vi "main 0.8.vi"() -> ()   [LabVIEW 2012]
uses:
  coherent/CH_LM/CH_LM Communication Mode.ctl
  ISEGNHQxxu/iseg NHQ VISA Control.ctl
  <vilib>/Utility/file.llb/Read From Spreadsheet File (DBL).vi
  <vilib>/Analysis/1siggen.llb/Ramp Pattern by Samples.vi
  <vilib>/Utility/file.llb/Write To Spreadsheet File (DBL).vi
  <vilib>/Utility/file.llb/Write To Spreadsheet File (string).vi
  <vilib>/Platform/browser.llb/Open URL in Default Browser (path).vi
  <vilib>/Analysis/NI_AALBase.lvlib
  coherent/CH_LM.lvlib
panel:
  out "x-y":u32
  in  "avg[t] acc[f]":bool=TRUE
  in  "frames":i32=1000
  in  "array size 2":i32
  in  "dark_load":bool
  in  "binning":dbl=4.0
  in  "exp time [s]":dbl=0.01
  in  "threshold":i32=110
  in  "dark?":bool=TRUE
  in  "count?":bool
  in  "array size":i32
  out "power noise-o-meter":dbl format="%.1g"
  out "signal noise-o-meter":dbl format="%.1g"
  in  "Nominal Voltage":sgl=50.0 max=4000 format="%.2f"
  in  "volt_set":bool
  in  "open base path":bool
  out "laser power":sgl[unit]=6.5658234e-09 format="%.3f"
  out "Actual Voltage":dbl[unit]=-50.050000000000004 format="%.2f"
  out "Waveform Chart":dbl(graph)
  in  "Path":path=path "Y:/Ediff/data/2016/10/161018"
  in  "stop":bool
  out "Slide":dbl(slide)=0.999 scale=0.0..1.0
  in  "Tab Control":T1(tab)
  in  "snap":bool
  in  "dark":bool
  in  "savebin":bool
  in  "savepng":bool
  out "meas_voltage":i32
  in  "header":string="PowerVoltScan1"
  in  "meas_start_power":bool
  out "meas_power":sgl[unit]=6.5658234e-09 format="%.3f"
  out "Slide 2":dbl(slide)=0.999 scale=0.0..1.0
  in  "meas_stop_volt":bool
  in  "meas_start_volt":bool
  in  "head":string="PowerVoltScan1"
  in  "volt_start":dbl format="%0.2f"
  in  "volt_end":dbl=1.0 format="%0.2f"
  in  "volt_samples":i32=128
  in  "move2com":bool
  in  "window2":dbl=10000.0 caption="+/- window" format="%#_6e"
  in  "steps2":u32=21 caption="steps"
  out "XY":dbl[][](graph)
  in  "meas_start_XY":bool
  in  "Axis2":string(combo)="4D Z"
  in  "Axis1":string(combo)="4D Z"
  in  "window1":dbl=10000.0 caption="+/- window" format="%#_6e"
  in  "steps1":u32=21 caption="steps"
  in  "meas_stop_XY":bool
  in  "showcom":bool
  in  "VISA ISEG":refnum<visa-resource-name>="COM6"
  in  "Channel (A)":enum16{"A", "B"}(ring)=enum."B"
  in  "IP address":string="172.24.192.135"
  out "error out":errorcluster
  out "coherent":errorcluster
  in  "volt_timeout":u32=6000
  in  "volt_threshold":sgl=2.0 max=4000 format="%.2f"
  out "captured":dbl[][](graph)
  out "live":dbl[][](graph)
  in  "close":bool
  # "%"
  # "Axis2"
  # "Axis1"
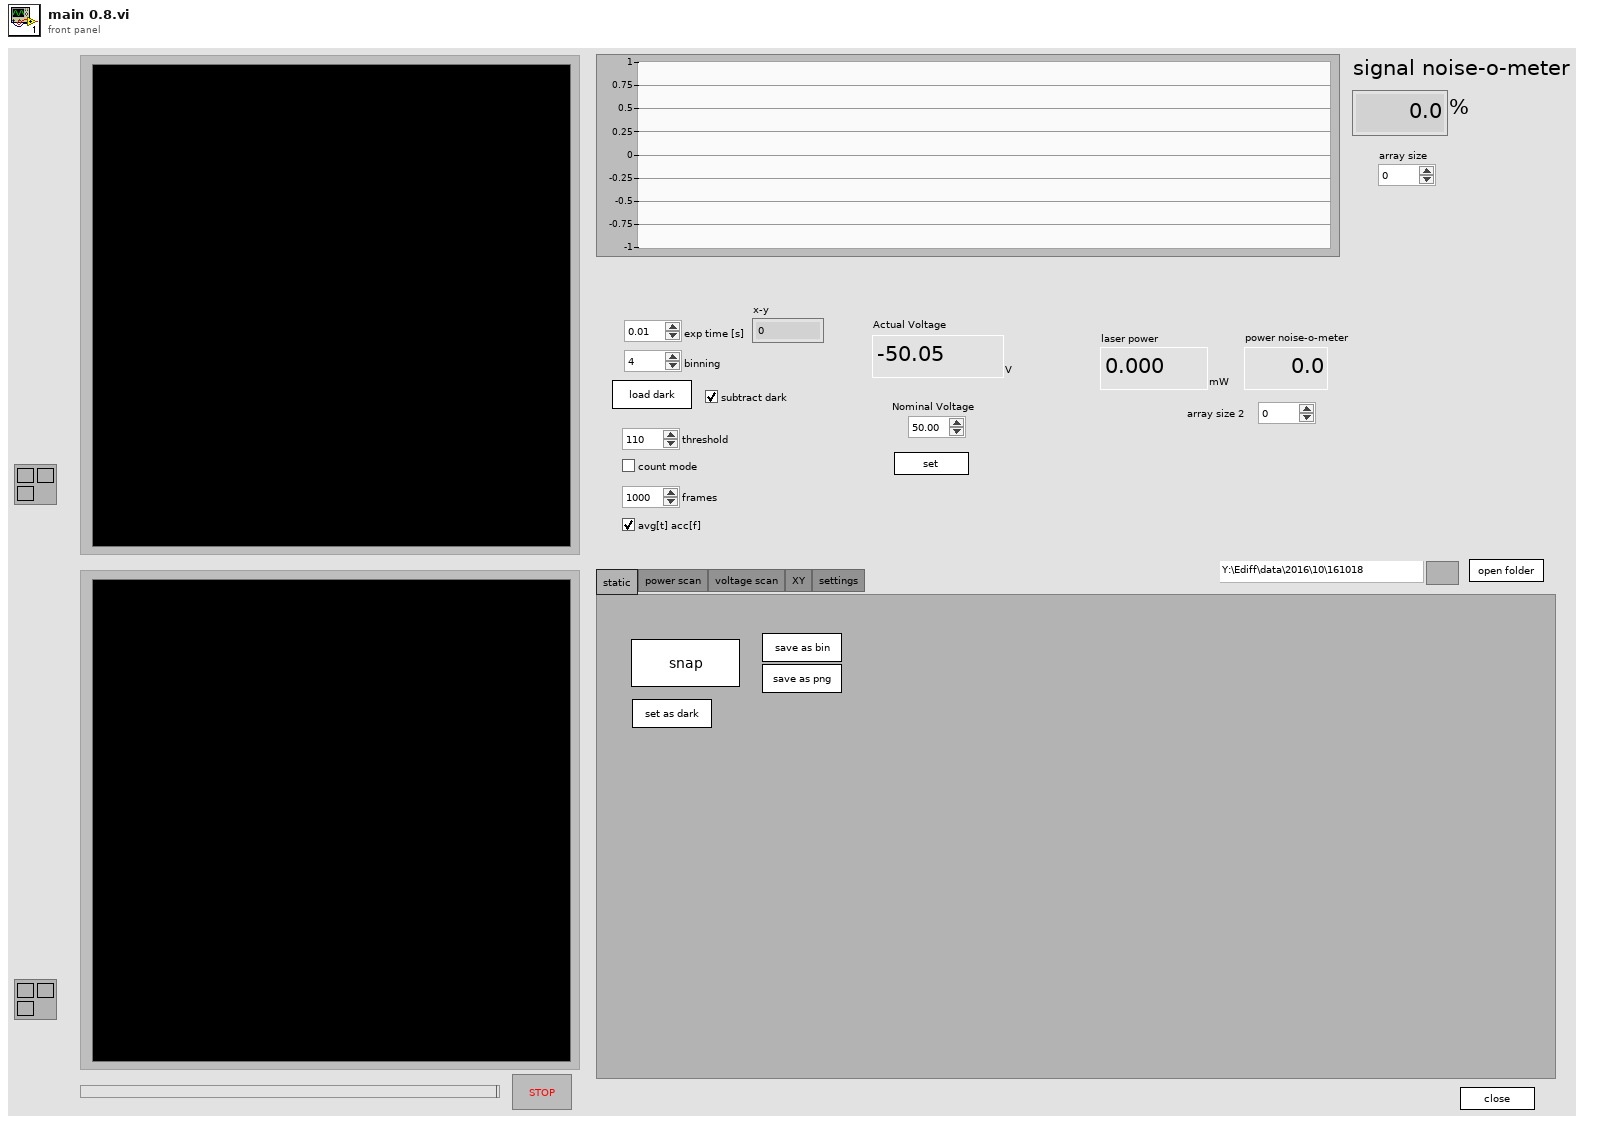
[diagram p1: front panel]
types:
  T1 = enum32{"static", "power scan", "voltage scan", "XY", "settings"}
  T2 = typedef "CH_LM.lvlib/CH_LM Communication Mode.ctl" = enum16{"None", "USB", "GPIB", "RS232"}
  T3 = typedef "Image Type" = u32
  T4 = typedef "IMAQ Image.ctl" = refnum<image>
  T5 = cluster{"height":u32, "width":u32, "datatype":u32}
  T6 = typedef "iseg NHQ VISA Control.ctl" = cluster{"VISA Resource Name":refnum<visa-resource-name>, "FP Notation":bool, "Maximum Voltage":u32, "Maximum Current":u32}
  T7 = typedef "CH_LM.lvlib/CH_LM Streaming Data.ctl" = cluster{"Value":sgl, "Quad Distance":cluster{"X":sgl, "Y":sgl}, "Display Data":cluster{"Format ID":u8, "Scale ID":u8}, "Unit ID":u8, "Flags":u32, "Pulse Period":u32, "Sequence ID":u32, "Unit String":string}
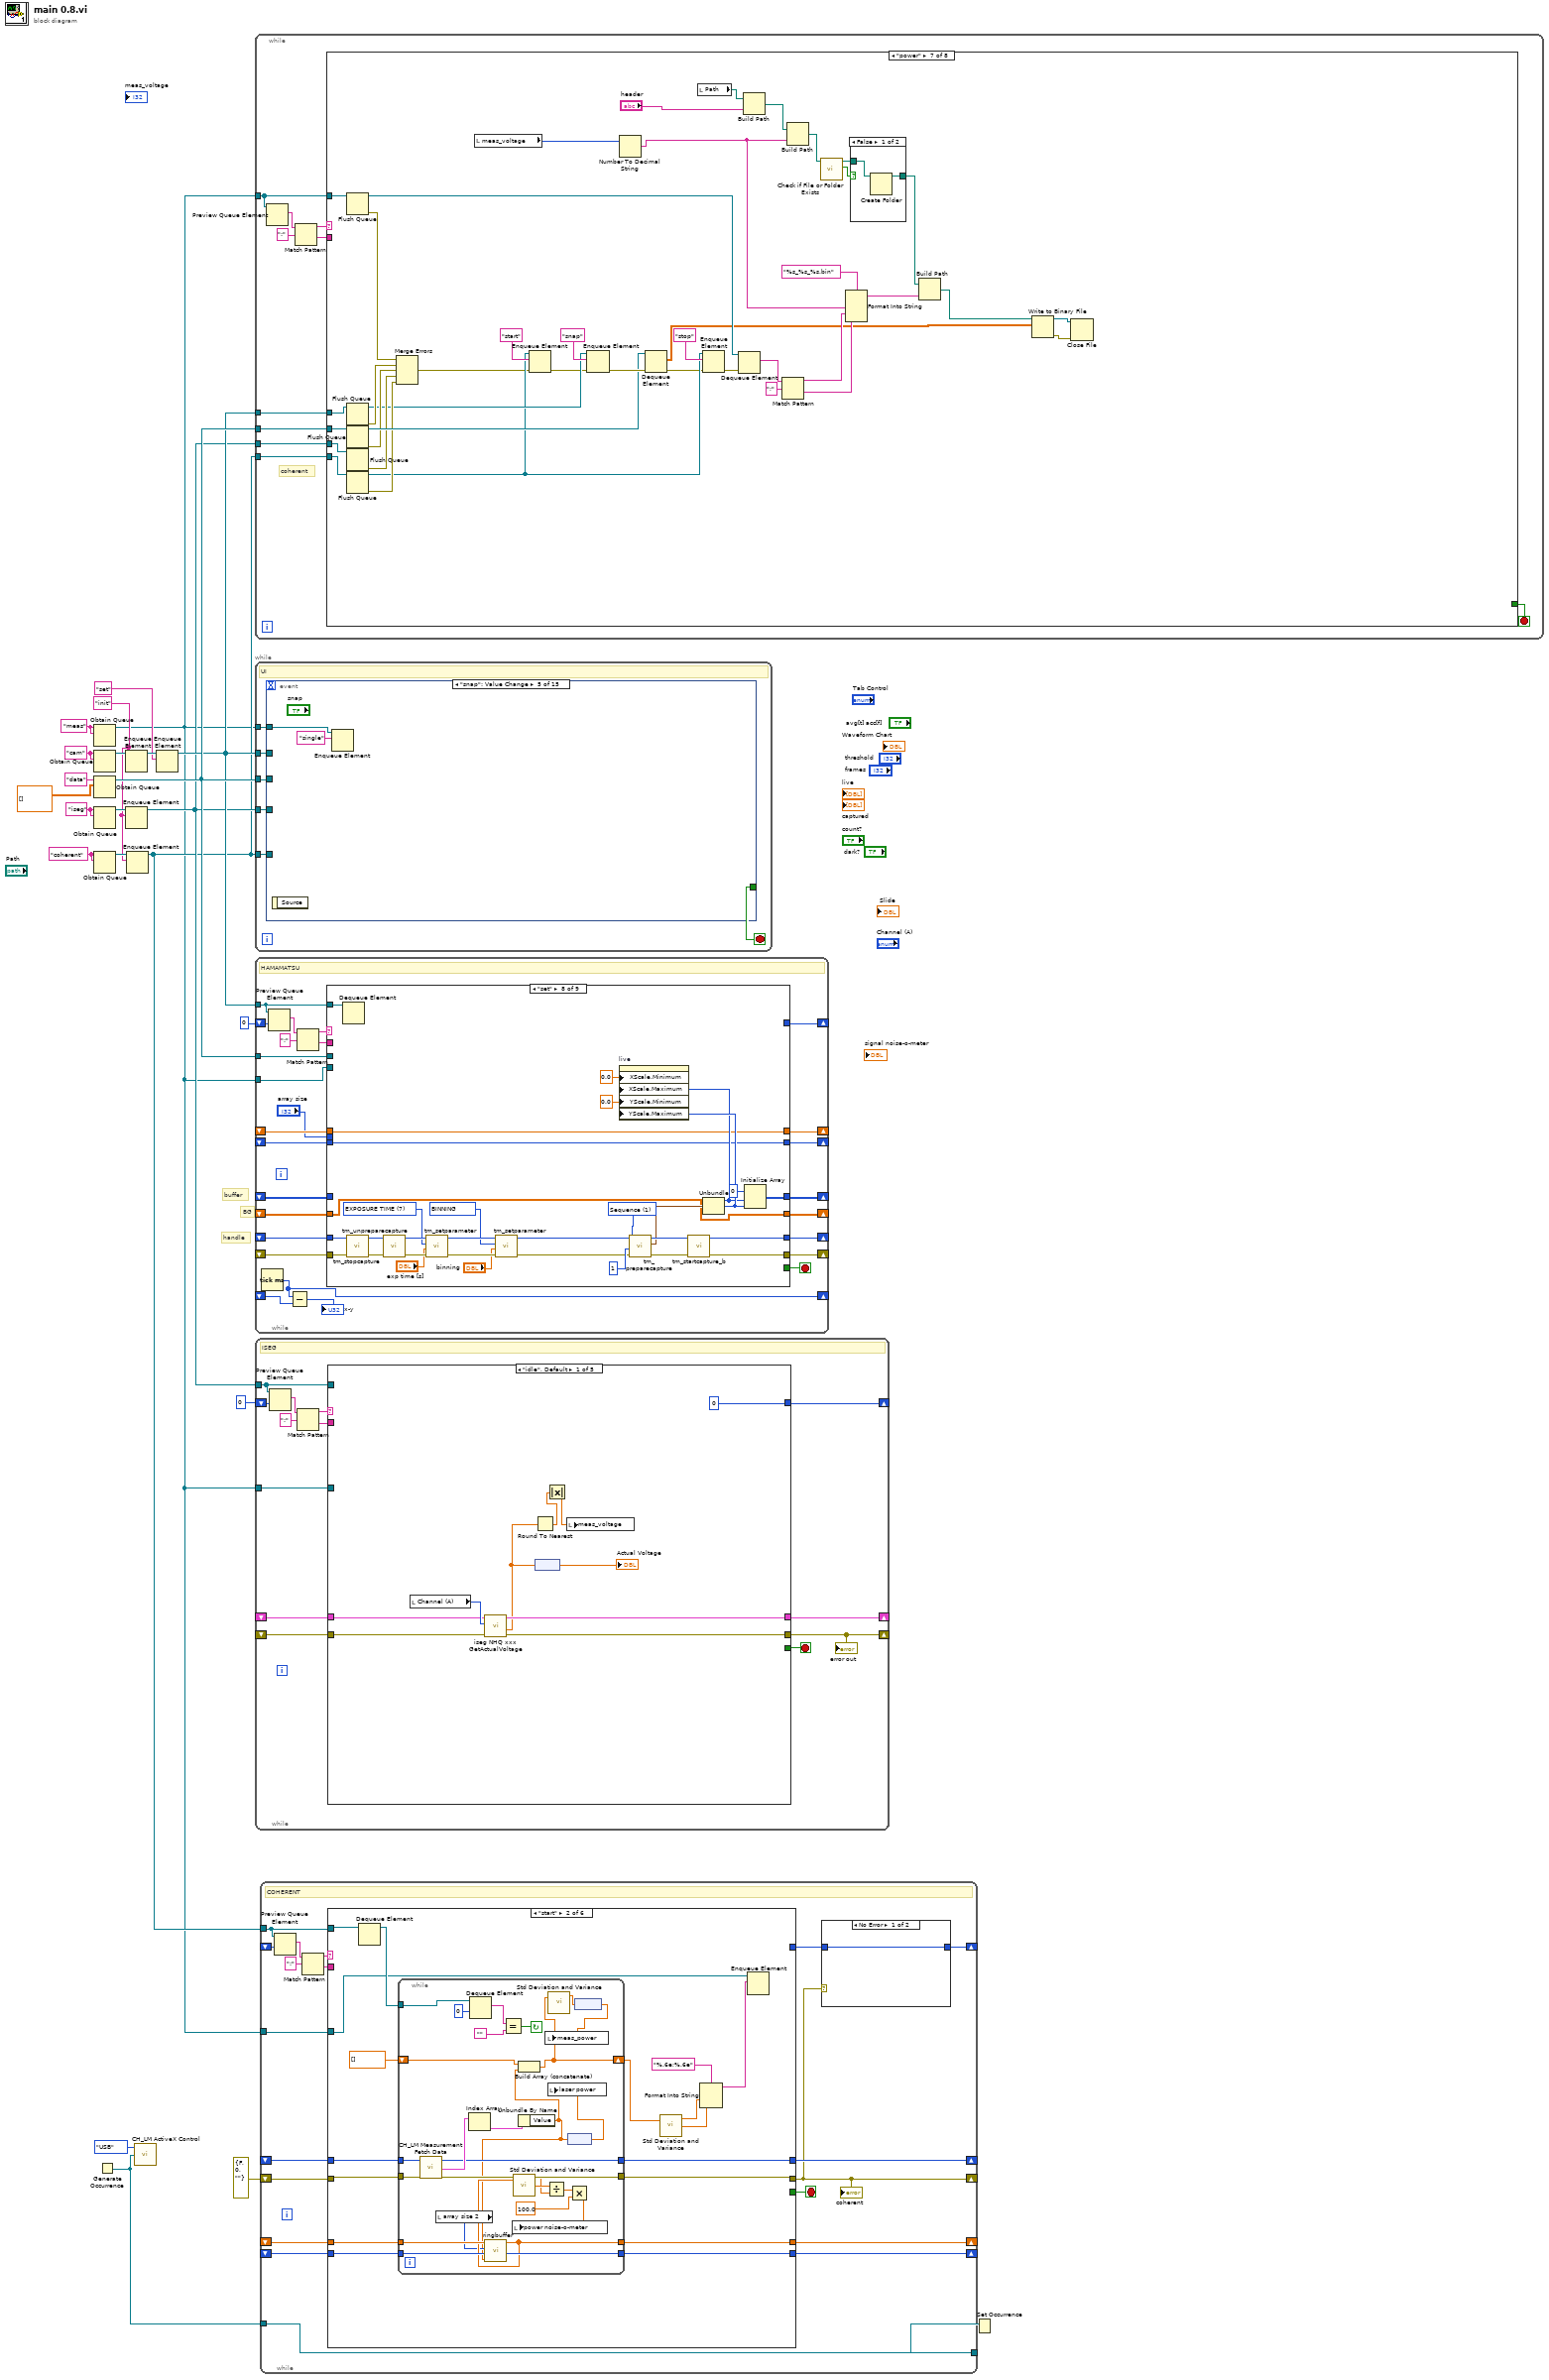
[diagram p0: block diagram]
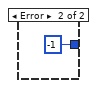
[diagram p2: hidden frame]
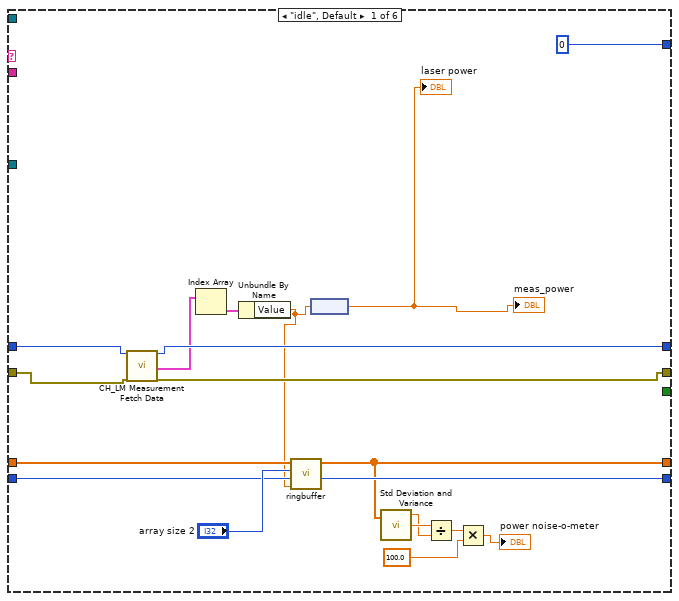
[diagram p3: hidden frame]
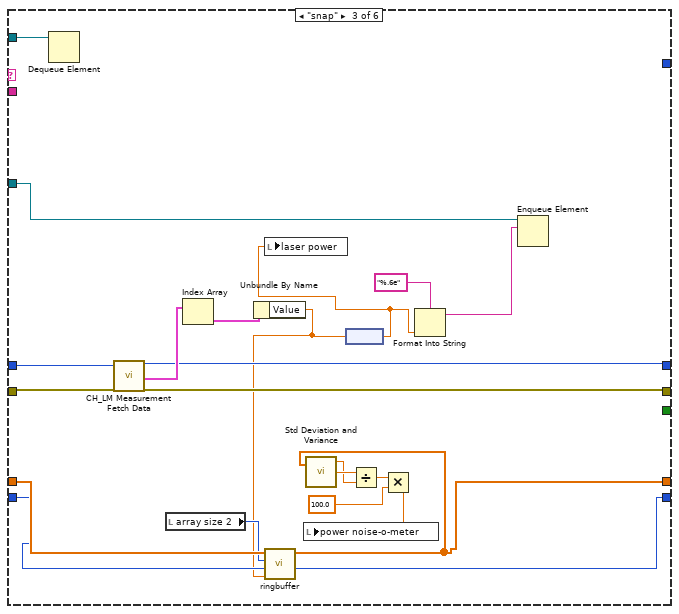
[diagram p4: hidden frame]
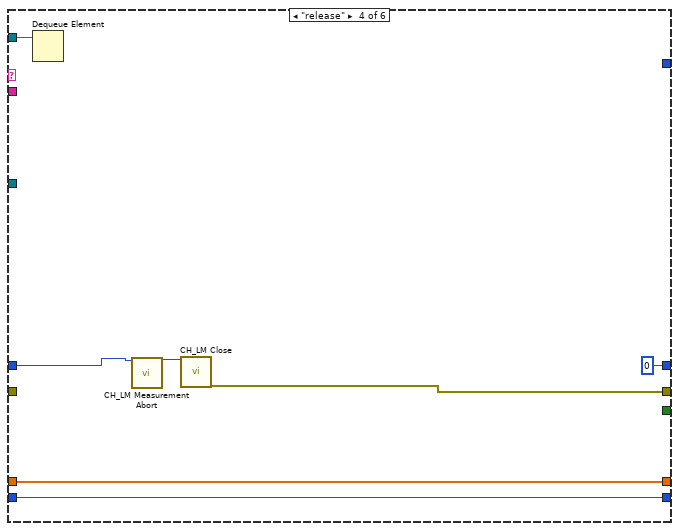
[diagram p5: hidden frame]
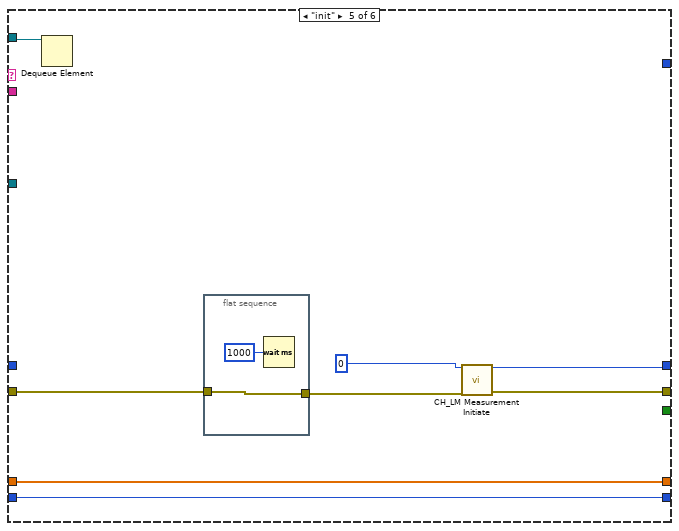
[diagram p6: hidden frame]
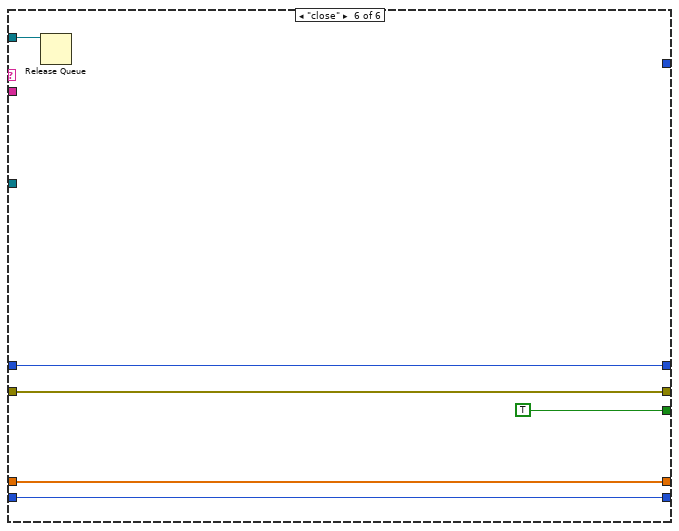
[diagram p7: hidden frame]
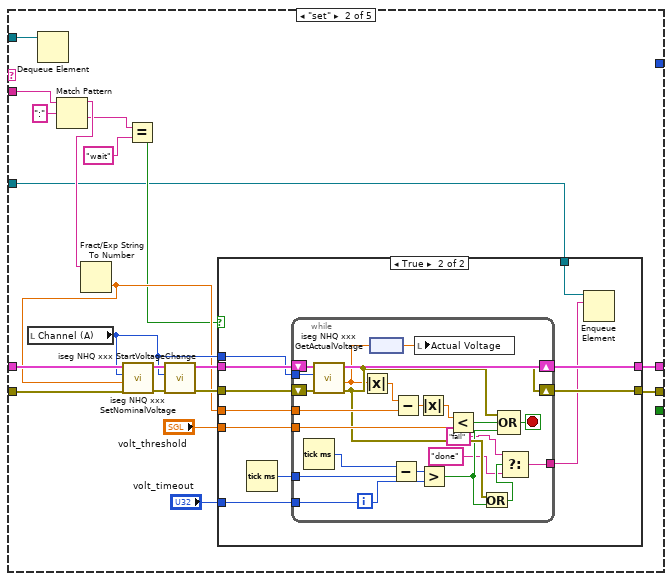
[diagram p8: hidden frame]
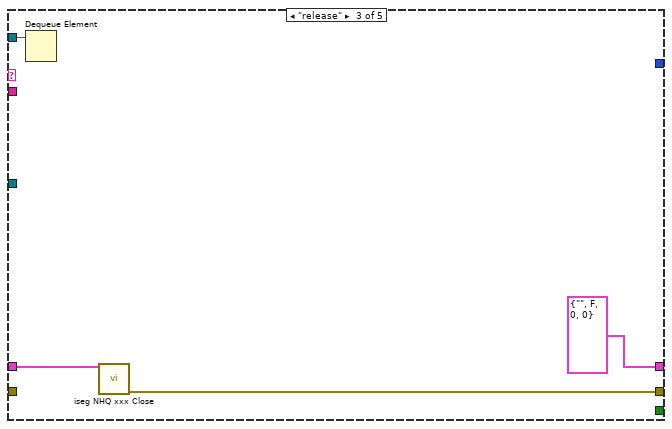
[diagram p10: hidden frame]
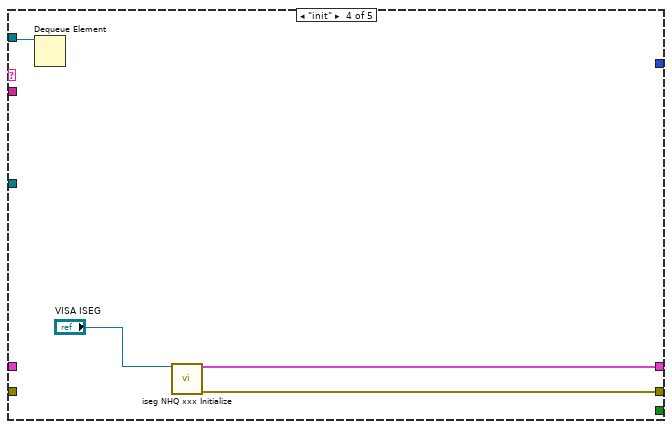
[diagram p11: hidden frame]
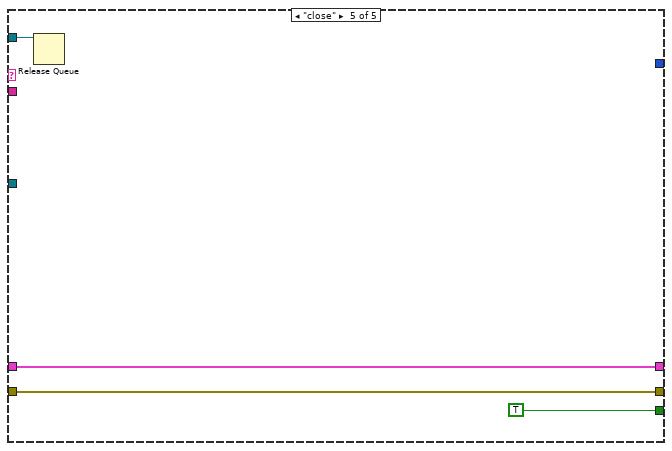
[diagram p12: hidden frame]
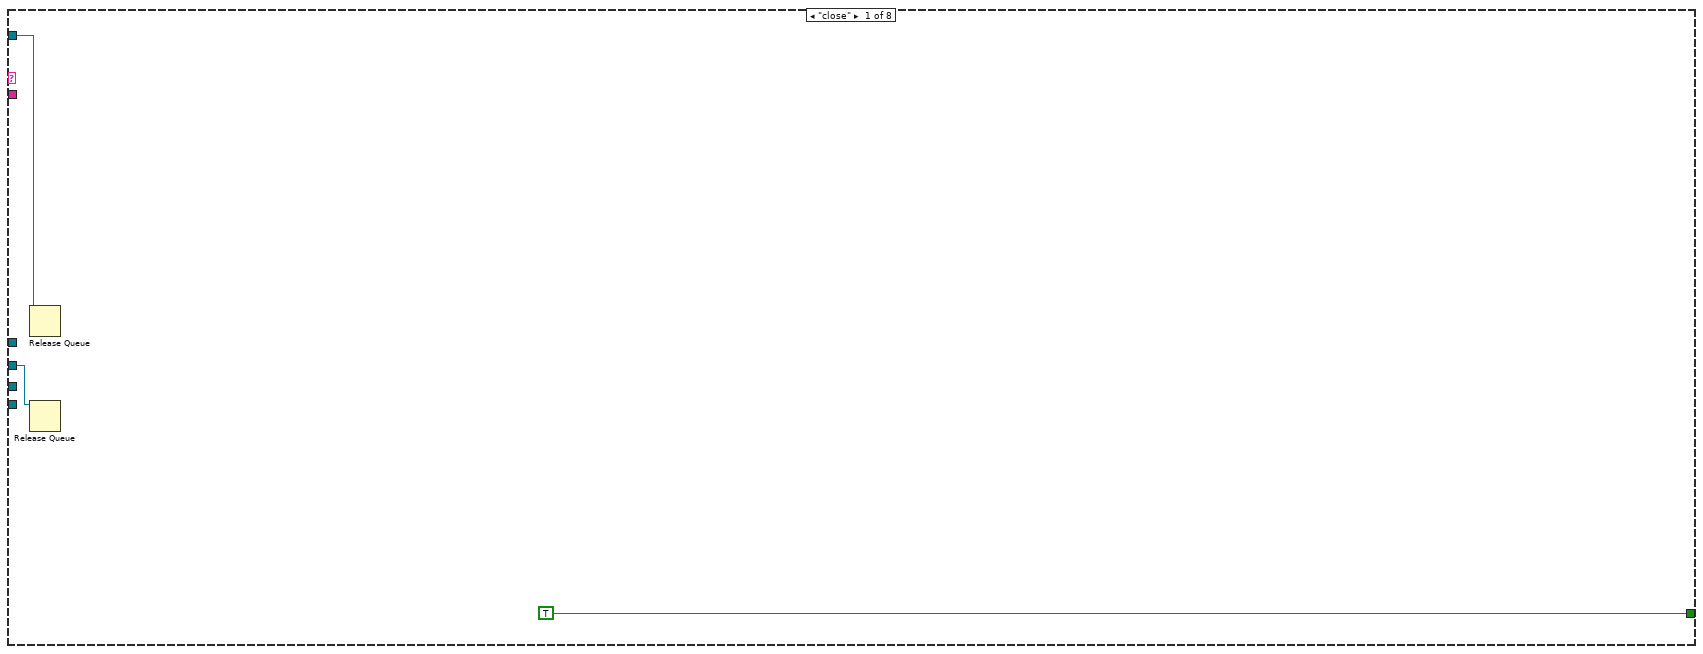
[diagram p13: hidden frame]
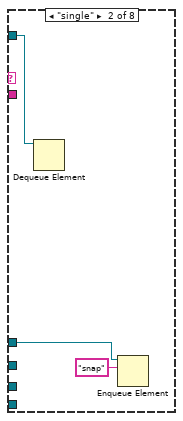
[diagram p14: hidden frame]
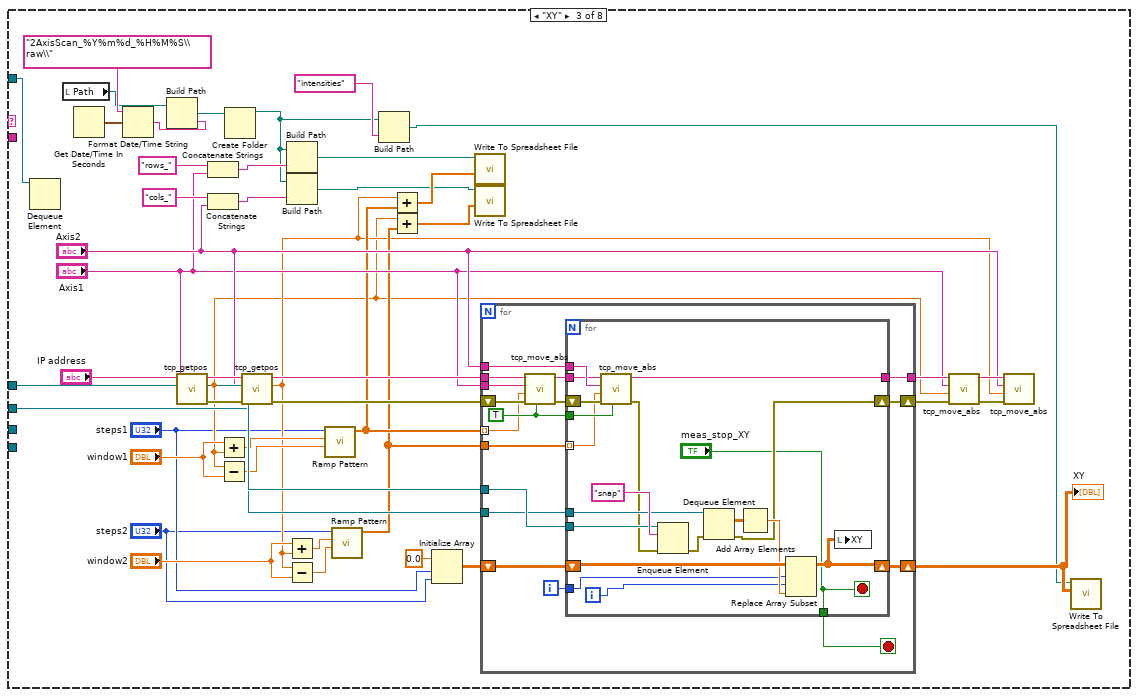
[diagram p15: hidden frame]
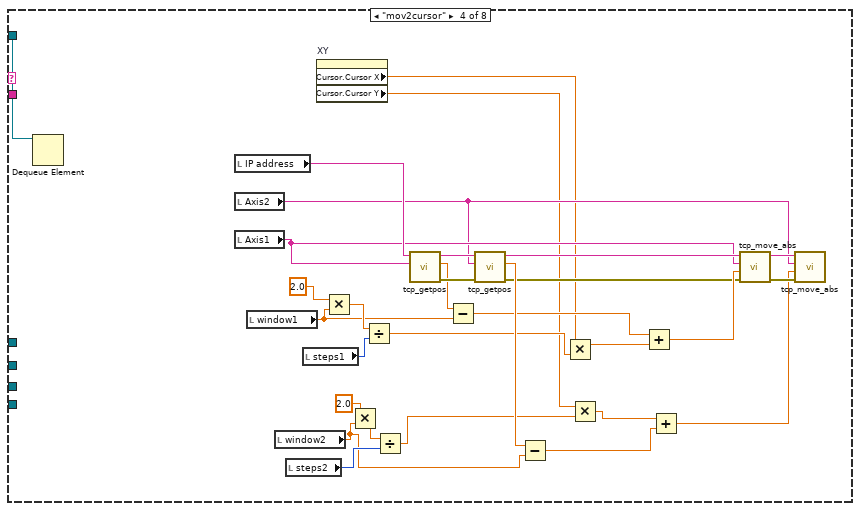
[diagram p16: hidden frame]
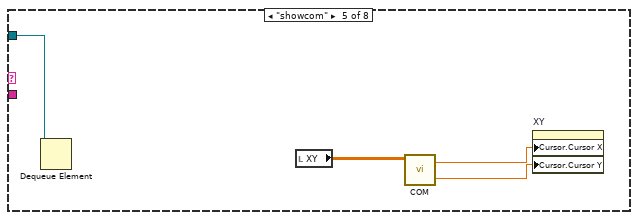
[diagram p17: hidden frame]
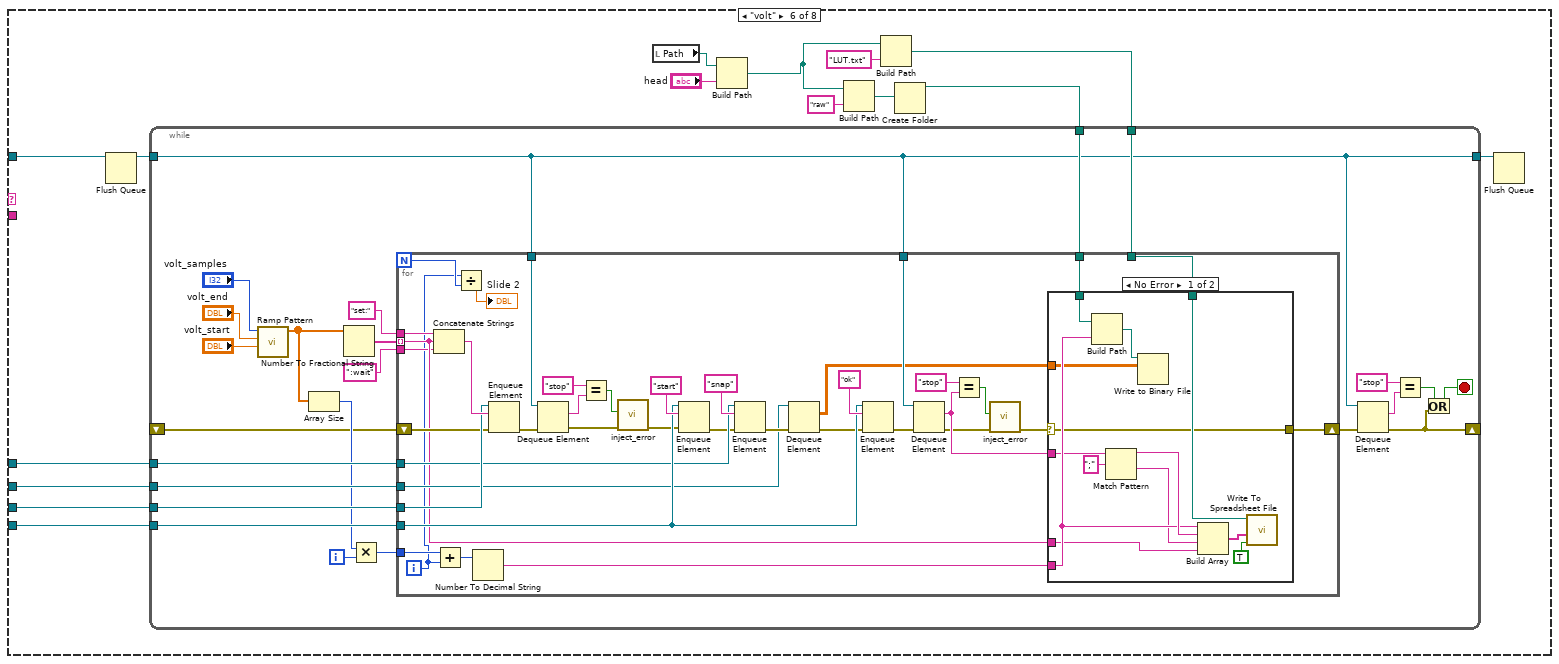
[diagram p18: hidden frame]
diagram:
  w8 = "coherent" ("name (unnamed)")
  w13 = "iseg" ("name (unnamed)")
  w7 = "init" ("element")
  w20 = "meas" ("name (unnamed)")
  w21 = "cam" ("name (unnamed)")
  # "BG"
  # "handle"
  # "buffer"
  n1 = Obtain Queue(name (unnamed)=w20, element data type=w20) -> (queue out=w1:refnum<queue>)  [unwired: 3 in, 2 out]
  n2 = Obtain Queue(name (unnamed)=w21, element data type=w21) -> (queue out=w23:refnum<queue>)  [unwired: 3 in, 2 out]
  n3 = Obtain Queue(name (unnamed)=w13, element data type=w13) -> (queue out=w12:refnum<queue>)  [unwired: 3 in, 2 out]
  n4 = Obtain Queue(name (unnamed)="data", element data type=dbl[][] []) -> (queue out=w16:refnum<queue>)  [unwired: 3 in, 2 out]
  n5 = Obtain Queue(name (unnamed)=w8, element data type=w8) -> (queue out=w9:refnum<queue>)  [unwired: 3 in, 2 out]
  n6 = Generate Occurrence() -> (w5:refnum<k4>)
  n7 = Enqueue Element(queue=w23, element=w7) -> (queue out=w19:refnum<queue>)  [unwired: 2 in, 2 out]
  n8 = Enqueue Element(queue=w12, element=w7) -> (queue out=w10:refnum<queue>)  [unwired: 2 in, 2 out]
  n9 = Enqueue Element(queue=w9, element=w7) -> (queue out=w3:refnum<queue>)  [unwired: 2 in, 2 out]
  n10 = call "CH_LM ActiveX Control.vi"("Communication Mode"=CH_LM_Communication_Mode."USB", "MonitorStop Occurrence"=w5) -> ()  [unwired: 3 in, 1 out]
  n11 = Enqueue Element(queue=w19, element="set") -> (queue out=w15:refnum<queue>)  [unwired: 2 in, 2 out]
  n12 = while {
    tunnel: w1 -> [w29]
    tunnel: w16 -> [w28]
    tunnel: w15 -> [w26]
    tunnel: w10 -> [w25]
    tunnel: w3 -> [w24]
    stop <- w27 stop-if-true
    # "coherent"
    n13 = Preview Queue Element(queue=w29) -> (element=w33:string)  [unwired: 2 in, 3 out]
    n14 = Match Pattern(string=w33, regular expression=":") -> (before substring=w31:string, after substring=w30:string)  [unwired: 1 in, 2 out]
    n15 = case shown="\"power\"" w31 {
      tunnel: w30 -> [_ _ _ _ _ _ _ _]
      tunnel: w29 -> [w35 w39 w84 w150 w151 w169 w285 _]
      tunnel: w28 -> [w36 _ w80 _ _ w161 w281 _]
      tunnel: [TRUE _ _ _ _ _ _ _] -> w27
      tunnel: w26 -> [_ w38 w81 _ _ w162 w279 _]
      tunnel: w25 -> [_ _ _ _ _ w163 w278 _]
      tunnel: w24 -> [_ _ _ _ _ w164 w277 _]
      frame "close" {
        n16 = Release Queue(queue=w35) -> ()  [unwired: 2 in, 3 out]
        n17 = Release Queue(queue=w36) -> ()  [unwired: 2 in, 3 out]
      }
      frame "single" {
        n18 = Dequeue Element(queue=w39) -> ()  [unwired: 2 in, 4 out]
        n19 = Enqueue Element(queue=w38, element="snap") -> ()  [unwired: 2 in, 3 out]
      }
      frame "XY" {
        n20 = Dequeue Element(queue=w84) -> ()  [unwired: 2 in, 4 out]
        n21 = local read "Path"() -> (w75:path)
        n22 = Get Date/Time In Seconds() -> (seconds since 1Jan1904=w79:timestamp)
        n23 = Format Date/Time String(time format string (%c)="2AxisScan_%Y%m%d_%H%M%S\\raw\\", seconds (now)=w79) -> (date/time string=w43:string)  [unwired: 1 in]
        n24 = Build Path(base path=w75, name or relative path=w43) -> (appended path=w47:path)
        n25 = call "tcp_getpos.vi"("Axis"="Axis1", "IP address"="IP address") -> ("error out"=w76:errorcluster, "position"=w52:dbl, "IP address out"=w77:string)  [unwired: 7 in]
        n26 = Concatenate Strings("rows_" ("string"), "Axis1") -> (w44:string)
        n27 = Concatenate Strings("cols_" ("string"), "Axis2") -> (w74:string)
        n28 = Add(x="window1", y=w52) -> (x+y=w59:dbl)
        n29 = Subtract(x=w52, y="window1") -> (x-y=w58:dbl)
        n30 = Create Folder(path (use dialog)=w47) -> (created path=w42:path)  [unwired: 2 in, 2 out]
        n31 = call "tcp_getpos.vi"("error in (no error)"=w76, "Axis"="Axis2", "IP address"=w77) -> ("error out"=w69:errorcluster, "position"=w53:dbl, "IP address out"=w64:string)  [unwired: 6 in]
        n32 = Build Path(base path=w42, name or relative path=w44) -> (appended path=w41:path)
        n33 = Build Path(base path=w42, name or relative path=w74) -> (appended path=w40:path)
        n34 = Add(x="window2", y=w53) -> (x+y=w56:dbl)
        n35 = Subtract(x=w53, y="window2") -> (x-y=w57:dbl)
        n36 = call-poly <vilib>:"Ramp Pattern.vi"("start"=w58, "end"=w59, "samples"="steps1") -> ("Ramp Pattern"=w55:dbl[])  [unwired: 7 in, 1 out]
        n37 = call-poly <vilib>:"Ramp Pattern.vi"("start"=w57, "end"=w56, "samples"="steps2") -> ("Ramp Pattern"=w54:dbl[])  [unwired: 7 in, 1 out]
        n38 = Build Path(base path=w42, name or relative path="intensities") -> (appended path=w45:path)
        n39 = Add(x=w53, y=w55) -> (x+y=w51:dbl[])
        n40 = Add(x=w52, y=w54) -> (x+y=w50:dbl[])
        n41 = Initialize Array(0.0 ("element"), "steps1", "steps2") -> (w82:dbl[][])
        n42 = call-poly <vilib>:"Write To Spreadsheet File.vi"("1D data"=w51, "file path (dialog if empty)"=w41) -> ()  [unwired: 6 in, 1 out]
        n43 = call-poly <vilib>:"Write To Spreadsheet File.vi"("1D data"=w50, "file path (dialog if empty)"=w40) -> ()  [unwired: 6 in, 1 out]
        n44 = for {
          tunnel: "Axis1" -> [w101]
          tunnel: w81 -> [w100]
          tunnel: w80 -> [w99]
          tunnel: "Axis2" -> [w95]
          shift-right: [w94] -> w73
          shift-left: w82 -> [w98]
          shift-right: [w91] -> w70
          shift-left: w69 -> [w90]
          tunnel: [w88] -> w65
          tunnel: w64 -> [w87]
          tunnel: w55 -> [w85] mode=indexing
          tunnel: w54 -> [w86]
          i -> [w97]
          stop <- w89 stop-if-true
          w96 = TRUE ("wait4motiondone")
          n45 = call "tcp_move_abs.vi"("wait4motiondone"=w96, "error in (no error)"=w90, "destination nm/u°"=w85, "Axis"=w101, "IP address"=w87) -> ("error out"=w93:errorcluster, "IP address out"=w92:string)  [unwired: 4 in, 1 out]
          n46 = for {
            tunnel: w100 -> [w118]
            tunnel: w99 -> [w117]
            tunnel: w97 -> [w103]
            shift-right: [w108] -> w94
            shift-left: w98 -> [w116]
            tunnel: w96 -> [w112]
            tunnel: w95 -> [w111]
            tunnel: w92 -> [w109]
            shift-right: [w107] -> w91
            shift-left: w93 -> [w110]
            tunnel: ["meas_stop_XY"] -> w89
            tunnel: [w105] -> w88
            tunnel: w86 -> [w104] mode=indexing
            i -> [w102]
            stop <- "meas_stop_XY" stop-if-true
            n47 = call "tcp_move_abs.vi"("wait4motiondone"=w112, "error in (no error)"=w110, "destination nm/u°"=w104, "Axis"=w111, "IP address"=w109) -> ("error out"=w113:errorcluster, "IP address out"=w105:string)  [unwired: 4 in, 1 out]
            n48 = Enqueue Element(queue=w118, element="snap", error in (no error)=w113) -> (error out=w119:errorcluster)  [unwired: 1 in, 2 out]
            n49 = Dequeue Element(queue=w117, error in (no error)=w119) -> (element=w115:dbl[][], error out=w107:errorcluster)  [unwired: 1 in, 2 out]
            n50 = Add Array Elements(numeric array=w115) -> (sum=w114:dbl)
            n51 = Replace Array Subset(array=w116, new element=w114, index (row)=w103, index (col)=w102) -> (w108:dbl[][])
            n52 = local write "XY"(w108) -> ()
          }
        }
        "XY" <- w73
        n53 = call "tcp_move_abs.vi"("error in (no error)"=w70, "destination nm/u°"=w52, "Axis"="Axis1", "IP address"=w65) -> ("error out"=w72:errorcluster, "IP address out"=w71:string)  [unwired: 5 in, 1 out]
        n54 = call "tcp_move_abs.vi"("error in (no error)"=w72, "destination nm/u°"=w53, "Axis"="Axis2", "IP address"=w71) -> ()  [unwired: 5 in, 3 out]
        n55 = call-poly <vilib>:"Write To Spreadsheet File.vi"("2D data"=w73, "file path (dialog if empty)"=w45) -> ()  [unwired: 6 in, 1 out]
      }
      frame "mov2cursor" {
        n56 = Dequeue Element(queue=w150) -> ()  [unwired: 2 in, 4 out]
        n57 = local read "IP address"() -> (w145:string)
        n58 = local read "Axis2"() -> (w123:string)
        n59 = local read "Axis1"() -> (w124:string)
        n60 = local read "window1"() -> (w138:dbl)
        n61 = local read "window2"() -> (w137:dbl)
        n62 = local read "steps2"() -> (w143:u32)
        n63 = local read "steps1"() -> (w144:u32)
        n64 = property on="XY" class="IntGraph (strict)"() -> ("Cursor.Cursor X"=w122:dbl, "Cursor.Cursor Y"=w121:dbl)  [unwired: 2 in, 2 out]
        n65 = Multiply(x=2.0, y=w138) -> (x*y=w142:dbl)
        n66 = Multiply(x=2.0, y=w137) -> (x*y=w139:dbl)
        n67 = Divide(x=w142, y=w144) -> (x/y=w136:dbl)
        n68 = Divide(x=w139, y=w143) -> (x/y=w133:dbl)
        n69 = call "tcp_getpos.vi"("Axis"=w124, "IP address"=w145) -> ("error out"=w148:errorcluster, "position"=w146:dbl, "IP address out"=w149:string)  [unwired: 7 in]
        n70 = Subtract(x=w146, y=w138) -> (x-y=w134:dbl)
        n71 = call "tcp_getpos.vi"("error in (no error)"=w148, "Axis"=w123, "IP address"=w149) -> ("error out"=w126:errorcluster, "position"=w147:dbl, "IP address out"=w125:string)  [unwired: 6 in]
        n72 = Subtract(x=w147, y=w137) -> (x-y=w131:dbl)
        n73 = Multiply(x=w122, y=w136) -> (x*y=w135:dbl)
        n74 = Multiply(x=w121, y=w133) -> (x*y=w132:dbl)
        n75 = Add(x=w134, y=w135) -> (x+y=w128:dbl)
        n76 = Add(x=w132, y=w131) -> (x+y=w127:dbl)
        n77 = call "tcp_move_abs.vi"("error in (no error)"=w126, "destination nm/u°"=w128, "Axis"=w124, "IP address"=w125) -> ("error out"=w130:errorcluster, "IP address out"=w129:string)  [unwired: 5 in, 1 out]
        n78 = call "tcp_move_abs.vi"("error in (no error)"=w130, "destination nm/u°"=w127, "Axis"=w123, "IP address"=w129) -> ()  [unwired: 5 in, 3 out]
      }
      frame "showcom" {
        n79 = Dequeue Element(queue=w151) -> ()  [unwired: 2 in, 4 out]
        n80 = local read "XY"() -> (w154:dbl[][])
        n81 = call "COM.vi"("Array"=w154) -> ("Y out"=w152:dbl, "X out"=w153:dbl)  [unwired: 3 in]
        n82 = property on="XY" class="IntGraph (strict)"("Cursor.Cursor X"=w153, "Cursor.Cursor Y"=w152) -> ()  [unwired: 2 in, 2 out]
      }
      frame "volt" {
        n83 = Flush Queue(queue=w169) -> (queue out=w165:refnum<queue>)  [unwired: 1 in, 2 out]
        n84 = local read "Path"() -> (w168:path)
        n85 = Build Path(base path=w168, name or relative path="head") -> (appended path=w156:path)
        n86 = Build Path(base path=w156, name or relative path="raw") -> (appended path=w158:path)
        n87 = Build Path(base path=w156, name or relative path="LUT.txt") -> (appended path=w159:path)
        n88 = Create Folder(path (use dialog)=w158) -> (created path=w157:path)  [unwired: 2 in, 2 out]
        n89 = while {
          tunnel: w165 -> [w170]
          tunnel: w164 -> [w193]
          tunnel: w163 -> [w187]
          tunnel: w162 -> [w186]
          tunnel: w161 -> [w185]
          tunnel: w159 -> [w180]
          tunnel: w157 -> [w179]
          shift-right: [w172] -> _
          shift-left: _ -> [w177]
          tunnel: [w170] -> w155
          i -> [w184]
          stop <- w171 stop-if-true
          n90 = call-poly <vilib>:"Ramp Pattern.vi"("start"="volt_start", "end"="volt_end", "samples"="volt_samples") -> ("Ramp Pattern"=w183:dbl[])  [unwired: 7 in, 1 out]
          n91 = Array Size(array=w183) -> (size(s)=w182:i32)
          n92 = Number To Fractional String(number=w183) -> (F-format string=w189:string[])  [unwired: 3 in]
          n93 = Multiply(x=w182, y=w184) -> (x*y=w181:i32)
          n94 = for {
            N -> [w196]
            tunnel: w193 -> [w223]
            tunnel: w170 -> [w230]
            tunnel: w189 -> [w213] mode=indexing
            tunnel: "set:" ("element") -> [w227]
            tunnel: w187 -> [w226]
            tunnel: w170 -> [w224]
            tunnel: w186 -> [w221]
            tunnel: w185 -> [w218]
            shift-right: [w198] -> w178
            shift-left: w177 -> [w216]
            tunnel: w181 -> [w215]
            tunnel: w180 -> [w212]
            tunnel: w179 -> [w211]
            tunnel: ":wait" ("element") -> [w197]
            i -> [w195]
            n95 = Concatenate Strings(w227, w213, w197) -> (w228:string)
            n96 = Add(x=w215, y=w195) -> (x+y=w214:i32)
            n97 = Divide(x=w195, y=w196) -> (x/y=→"Slide 2":dbl)
            n98 = Number To Decimal String(number=w214) -> (decimal integer string=w210:string)  [unwired: 1 in]
            n99 = Enqueue Element(queue=w226, element=w228, error in (no error)=w216) -> (error out=w225:errorcluster)  [unwired: 1 in, 2 out]
            n100 = Dequeue Element(queue=w224, error in (no error)=w225) -> (element=w207:string, error out=w205:errorcluster)  [unwired: 1 in, 2 out]
            n101 = Equal?(x="stop" ("y"), y=w207) -> (x = y?=w204:bool)
            n102 = call "inject_error.vi"("error in"=w205, "s"=w204) -> ("error out"=w206:errorcluster)  [unwired: 9 in]
            n103 = Enqueue Element(queue=w223, element="start", error in (no error)=w206) -> (error out=w220:errorcluster)  [unwired: 1 in, 2 out]
            n104 = Enqueue Element(queue=w221, element="snap", error in (no error)=w220) -> (error out=w219:errorcluster)  [unwired: 1 in, 2 out]
            n105 = Dequeue Element(queue=w218, error in (no error)=w219) -> (element=w209:dbl[][], error out=w217:errorcluster)  [unwired: 1 in, 2 out]
            n106 = Enqueue Element(queue=w223, element="ok", error in (no error)=w217) -> (error out=w229:errorcluster)  [unwired: 1 in, 2 out]
            n107 = Dequeue Element(queue=w230, error in (no error)=w229) -> (element=w201:string, error out=w200:errorcluster)  [unwired: 1 in, 2 out]
            n108 = Equal?(x="stop" ("y"), y=w201) -> (x = y?=w203:bool)
            n109 = call "inject_error.vi"("error in"=w200, "s"=w203) -> ("error out"=w199:errorcluster)  [unwired: 9 in]
            n110 = case shown="No Error" w199 {
              selector: w199 -> [w235 w246]
              tunnel: w213 -> [w234 _]
              tunnel: w212 -> [w241 _]
              tunnel: w211 -> [w240 _]
              tunnel: w210 -> [w239 _]
              tunnel: w209 -> [w237 _]
              tunnel: w201 -> [w236 _]
              tunnel: [w235 w246] -> w198
              frame No Error {
                n111 = Build Path(base path=w240, name or relative path=w239) -> (appended path=w238:path)
                n112 = Match Pattern(string=w236, regular expression=";") -> (before substring=w243:string, after substring=w233:string)  [unwired: 1 in, 2 out]
                n113 = Write to Binary File(file (use dialog)=w238, data=w237) -> ()  [unwired: 4 in, 3 out]
                n114 = Build Array(w239, w243, w233, w234) -> (w242:string[])
                n115 = call-poly <vilib>:"Write To Spreadsheet File.vi"("append to file? (new file:F)"=TRUE, "1D data"=w242, "file path (dialog if empty)"=w241) -> ()  [unwired: 5 in, 1 out]
              }
              frame Error {
              }
            }
          }
          n116 = Dequeue Element(queue=w170, error in (no error)=w178) -> (element=w175:string, error out=w172:errorcluster)  [unwired: 1 in, 2 out]
          n117 = Equal?(x="stop" ("y"), y=w175) -> (x = y?=w173:bool)
          n118 = Or(x=w173, y=w172) -> (x .or. y?=w171:bool)
        }
        n119 = Flush Queue(queue=w155) -> ()  [unwired: 1 in, 3 out]
      }
      frame "power" {
        n120 = Flush Queue(queue=w285) -> (queue out=w264:refnum<queue>, error out=w276:errorcluster)  [unwired: 1 in, 1 out]
        n121 = Flush Queue(queue=w279) -> (queue out=w271:refnum<queue>, error out=w275:errorcluster)  [unwired: 1 in, 1 out]
        n122 = Flush Queue(queue=w281) -> (queue out=w280:refnum<queue>, error out=w274:errorcluster)  [unwired: 1 in, 1 out]
        n123 = Flush Queue(queue=w278) -> (error out=w273:errorcluster)  [unwired: 1 in, 2 out]
        n124 = Flush Queue(queue=w277) -> (queue out=w268:refnum<queue>, error out=w272:errorcluster)  [unwired: 1 in, 1 out]
        n125 = Merge Errors(w276, w275, w274, w273, w272) -> (w265:errorcluster)
        n126 = local read "meas_voltage"() -> (w253:i32)
        n127 = Enqueue Element(queue=w268, element="start", error in (no error)=w265) -> (error out=w266:errorcluster)  [unwired: 1 in, 2 out]
        n128 = Enqueue Element(queue=w271, element="snap", error in (no error)=w266) -> (error out=w282:errorcluster)  [unwired: 1 in, 2 out]
        n129 = Number To Decimal String(number=w253) -> (decimal integer string=w259:string)  [unwired: 1 in]
        n130 = Dequeue Element(queue=w280, error in (no error)=w282) -> (element=w256:dbl[][], error out=w267:errorcluster)  [unwired: 1 in, 2 out]
        n131 = local read "Path"() -> (w287:path)
        n132 = Enqueue Element(queue=w268, element="stop", error in (no error)=w267) -> (error out=w263:errorcluster)  [unwired: 1 in, 2 out]
        n133 = Dequeue Element(queue=w264, error in (no error)=w263) -> (element=w261:string)  [unwired: 1 in, 3 out]
        n134 = Build Path(base path=w287, name or relative path="header") -> (appended path=w284:path)
        n135 = Match Pattern(string=w261, regular expression=";") -> (before substring=w258:string, after substring=w257:string)  [unwired: 1 in, 2 out]
        n136 = Build Path(base path=w284, name or relative path=w259) -> (appended path=w249:path)
        n137 = call <vilib>:"Check if File or Folder Exists.vi"("path"=w249) -> ("file or folder exists?"=w248:bool, "dup path"=w247:path)  [unwired: 8 in, 1 out]
        n138 = Format Into String(format string="%s_%s_%s.bin", w259, w258, w257) -> (resulting string=w255:string)  [unwired: 2 in, 1 out]
        n139 = case shown="False" w248 {
          tunnel: [w289 w290] -> w250
          tunnel: w247 -> [w288 w290]
          frame False {
            n140 = Create Folder(path (use dialog)=w288) -> (created path=w289:path)  [unwired: 2 in, 2 out]
          }
          frame True {
          }
        }
        n141 = Build Path(base path=w250, name or relative path=w255) -> (appended path=w254:path)
        n142 = Write to Binary File(file (use dialog)=w254, data=w256) -> (refnum out=w252:refnum<file>, error out=w251:errorcluster)  [unwired: 4 in, 1 out]
        n143 = Close File(refnum=w252, error in=w251) -> ()  [unwired: 2 out]
      }
      frame "idle", Default {
      }
    }
  }
  n144 = while {
    tunnel: w15 -> [w296]
    tunnel: w1 -> [w295]
    tunnel: w16 -> [w294]
    tunnel: w10 -> [w292]
    tunnel: w3 -> [w291]
    stop <- w293 stop-if-true
    # "UI"
    n145 = event shown="[4] \"snap\": Value Change" {
      selector: _ -> [_ _ _ _ _ _ _ _ _ _ _ _ _ _ _]
      dyn-events: _ -> [_ _ _ _ _ _ _ _ _ _ _ _ _ _ _]
      timeout: _ -> [_ _ _ _ _ _ _ _ _ _ _ _ _ _ _]
      tunnel: w296 -> [_ w305 w308 w310 _ _ _ _ _ _ _ w363 _ _ _]
      tunnel: w295 -> [_ w306 _ _ w311 w314 w315 w318 _ _ w357 _ w370 w372 _]
      tunnel: w294 -> [_ _ _ _ _ _ _ _ _ _ _ _ _ _ _]
      tunnel: [_ TRUE _ _ _ _ _ _ _ _ _ _ _ _ _] -> w293
      tunnel: w292 -> [_ w302 _ _ _ _ _ _ _ _ _ _ _ _ w377]
      tunnel: w291 -> [_ w299 _ _ _ _ _ _ _ _ _ _ _ _ _]
      event Timeout {
        n146 = event-data() -> ()  [unwired: 1 in, 1 out]
      }
      event "close": Value Change {
        w297 = "close" ("element")
        w298 = "release" ("element")
        n147 = event-data() -> ()  [unwired: 1 in, 1 out]
        n148 = Enqueue Element(queue=w299, element=w298) -> (queue out=w300:refnum<queue>)  [unwired: 2 in, 2 out]
        n149 = Enqueue Element(queue=w302, element=w298) -> (queue out=w301:refnum<queue>)  [unwired: 2 in, 2 out]
        n150 = Enqueue Element(queue=w305, element=w298) -> (queue out=w304:refnum<queue>)  [unwired: 2 in, 2 out]
        n151 = Enqueue Element(queue=w300, element=w297) -> ()  [unwired: 2 in, 3 out]
        n152 = Enqueue Element(queue=w301, element=w297) -> ()  [unwired: 2 in, 3 out]
        n153 = Enqueue Element(queue=w306, element=w297) -> ()  [unwired: 2 in, 3 out]
        n154 = Enqueue Element(queue=w304, element=w297) -> ()  [unwired: 2 in, 3 out]
      }
      event "dark": Value Change {
        n155 = event-data() -> ()  [unwired: 1 in, 1 out]
        n156 = Enqueue Element(queue=w308, element="dark") -> ()  [unwired: 2 in, 3 out]
      }
      event "binning", "exp time [s]": Value Change {
        n157 = event-data() -> ()  [unwired: 1 in, 1 out]
        n158 = Enqueue Element(queue=w310, element="set") -> ()  [unwired: 2 in, 3 out]
      }
      event "snap": Value Change {
        n159 = event-data() -> ()  [unwired: 1 in, 1 out]
        n160 = Enqueue Element(queue=w311, element="single") -> ()  [unwired: 2 in, 3 out]
      }
      event "meas_start_volt": Value Change {
        n161 = event-data() -> ()  [unwired: 1 in, 1 out]
        n162 = Enqueue Element(queue=w314, element="volt") -> ()  [unwired: 2 in, 3 out]
      }
      event "meas_stop_volt": Value Change {
        n163 = event-data() -> ()  [unwired: 1 in, 1 out]
        n164 = Enqueue Element(queue=w315, element="stop") -> ()  [unwired: 2 in, 3 out]
      }
      event "meas_start_power": Value Change {
        n165 = event-data() -> ()  [unwired: 1 in, 1 out]
        n166 = Enqueue Element(queue=w318, element="power") -> ()  [unwired: 2 in, 3 out]
      }
      event "open base path": Value Change {
        n167 = event-data() -> ()  [unwired: 1 in, 1 out]
        n168 = local read "Path"() -> (w319:path)
        n169 = call-poly <vilib>:"Open URL in Default Browser.vi"("path"=w319) -> ()  [unwired: 5 in, 2 out]
      }
      event "savebin", "savepng": Value Change {
        n170 = event-data() -> ()  [unwired: 1 in, 1 out]
        n171 = Get Date/Time In Seconds() -> (seconds since 1Jan1904=w325:timestamp)
        n172 = local read "Path"() -> (w321:path)
        n173 = Format Date/Time String(time format string (%c)="MCPIMG_%Y%m%d_%H%M%S", seconds (now)=w325) -> (date/time string=w320:string)  [unwired: 1 in]
        n174 = local read "captured"() -> (w322:dbl[][])
        n175 = case shown="False" "savebin" {
          tunnel: w322 -> [w340 w356]
          tunnel: w321 -> [w337 w350]
          tunnel: w320 -> [w335 w351]
          frame False {
            w345 = T3 7 items=["Grayscale (U8)", "Grayscale (I16)", "Grayscale (SGL)", "Complex (CSG)", "RGB (U32)", "HSL (U32)", "RGB (U64)", "Grayscale (U16)"] ("Image Type")
            n176 = for {
              tunnel: w340 -> [w348] mode=indexing
              tunnel: [w347] -> w339 mode=indexing
              n177 = Reverse 1D Array(array=w348) -> (reversed array=w347:dbl[])
            }
            n178 = Concatenate Strings(w335, ".png" ("string")) -> (w336:string)
            n179 = Transpose 2D Array(2D array=w339) -> (transposed array=w328:dbl[][])
            n180 = Array Max & Min(array=w328) -> (min value=w327:dbl)  [unwired: 3 out]
            n181 = Build Path(base path=w337, name or relative path=w336) -> (appended path=w338:path)
            n182 = Subtract(x=w328, y=w327) -> (x-y=w326:dbl[][])
            n183 = call "IMAQ Create"("Image Name"="untitled", "Image Type"=w345) -> ("New Image"=w346:T4)  [unwired: 3 in, 1 out]
            n184 = Array Max & Min(array=w326) -> (max value=w333:dbl)  [unwired: 3 out]
            n185 = Divide(x=w326, y=w333) -> (x/y=w332:dbl[][])
            n186 = Multiply(x=w332, y=255) -> (x*y=w330:dbl[][])
            n187 = To Unsigned Word Integer(number=w330) -> (unsigned 16bit integer=w329:u16[][])
            n188 = call "IMAQ ArrayToImage"("Image Pixels (U16)"=w329, "Image"=w346) -> ("Image Out"=w344:T4)  [unwired: 8 in, 1 out]
            n189 = call-poly "IMAQ Write File 2"("Image Quality"=u32 1000, "File Path"=w338, "Image"=w344) -> ("Image Out (duplicate)"=w342:T4)  [unwired: 7 in, 1 out]
            n190 = call "IMAQ Dispose"("Image"=w342) -> ()  [unwired: 5 in, 1 out]
          }
          frame True {
            n191 = Concatenate Strings(w351, ".bin" ("string")) -> (w353:string)
            n192 = Build Path(base path=w350, name or relative path=w353) -> (appended path=w349:path)
            n193 = Write to Binary File(file (use dialog)=w349, data=w356) -> (refnum out=w355:refnum<file>, error out=w354:errorcluster)  [unwired: 4 in, 1 out]
            n194 = Close File(refnum=w355, error in=w354) -> ()  [unwired: 2 out]
          }
        }
      }
      event "meas_start_XY": Value Change {
        n195 = event-data() -> ()  [unwired: 1 in, 1 out]
        n196 = Enqueue Element(queue=w357, element="XY") -> ()  [unwired: 2 in, 3 out]
      }
      event "dark_load": Value Change {
        n197 = event-data() -> ()  [unwired: 1 in, 1 out]
        n198 = local read "Path"() -> (w362:path)
        n199 = call "File Dialog"("start path"=w362) -> ("selected path"=w360:path, "cancelled"=w359:bool)  [unwired: 11 in, 2 out]
        n200 = case shown="False" w359 {
          tunnel: w363 -> [w368 _]
          tunnel: "dark_load:" ("element") -> [w366 _]
          tunnel: w360 -> [w364 _]
          frame False {
            n201 = Path To String(path=w364) -> (string=w365:string)
            n202 = Concatenate Strings(w366, w365) -> (w367:string)
            n203 = Enqueue Element(queue=w368, element=w367) -> ()  [unwired: 2 in, 3 out]
          }
          frame True {
          }
        }
      }
      event "move2com": Value Change {
        n204 = event-data() -> ()  [unwired: 1 in, 1 out]
        n205 = Enqueue Element(queue=w370, element="mov2cursor") -> ()  [unwired: 2 in, 3 out]
      }
      event "showcom": Value Change {
        n206 = event-data() -> ()  [unwired: 1 in, 1 out]
        n207 = Enqueue Element(queue=w372, element="showcom") -> ()  [unwired: 2 in, 3 out]
      }
      event "volt_set": Value Change {
        n208 = event-data() -> ()  [unwired: 1 in, 1 out]
        n209 = Number To Fractional String(number="Nominal Voltage") -> (F-format string=w373:string)  [unwired: 3 in]
        n210 = Concatenate Strings("set:" ("element"), w373) -> (w376:string)
        n211 = Enqueue Element(queue=w377, element=w376) -> ()  [unwired: 2 in, 3 out]
      }
    }
  }
  n212 = while {
    tunnel: w15 -> [w399]
    shift-right: [w397] -> _
    shift-left: _ -> [w396]
    shift-right: [w395] -> _
    shift-left: _ -> [w394]
    shift-right: [w393] -> _
    shift-left: _ -> [w392]
    shift-right: [w391] -> _
    shift-left: _ -> [w390]
    shift-right: [w388] -> _
    shift-left: 0 -> [w389]
    tunnel: w16 -> [w387]
    tunnel: w1 -> [w386]
    shift-right: [w385] -> _
    shift-left: _ -> [w384]
    shift-right: [w382] -> _
    shift-left: _ -> [w383]
    shift-right: [w379] -> _
    shift-left: _ -> [w380]
    stop <- w398 stop-if-true
    # "HAMAMATSU"
    n213 = Tick Count (ms)() -> (millisecond timer value=w379:u32)
    n214 = Preview Queue Element(queue=w399, timeout in ms (-1)=w389) -> (element=w403:string)  [unwired: 1 in, 3 out]
    n215 = Subtract(x=w379, y=w380) -> (x-y=→"x-y":u32)
    n216 = Match Pattern(string=w403, regular expression=":") -> (before substring=w401:string, after substring=w400:string)  [unwired: 1 in, 2 out]
    n217 = case shown="\"set\"" w401 {
      tunnel: w400 -> [_ _ _ _ w562 _ _ _ _]
      tunnel: w399 -> [_ w442 w507 w556 w566 w578 w581 w600 w626]
      tunnel: [_ _ _ _ _ _ _ _ TRUE] -> w398
      tunnel: [w422 w444 w512 w554 w563 w570 w586 w588 w621] -> w397
      tunnel: w396 -> [w424 w447 w514 w554 w563 w574 _ w618 w621]
      tunnel: [w423 w439 w511 w553 w564 u32 0 ("Handle out") w584 w589 w622] -> w395
      tunnel: w394 -> [w425 w445 w515 w553 w564 w575 _ w616 w622]
      tunnel: [w421 w446 w510 w555 w565 w576 w582 w601 w623] -> w393
      tunnel: w392 -> [w421 w446 w510 w555 w565 w576 w582 _ w623]
      tunnel: [w420 w443 w513 w552 w559 w577 w583 w592 w624] -> w391
      tunnel: w390 -> [w420 w443 w513 _ _ w577 w583 w592 w624]
      tunnel: [0 _ _ _ _ _ _ _ _] -> w388
      tunnel: w387 -> [_ w438 _ _ _ _ _ _ _]
      tunnel: w386 -> [_ _ w508 _ _ _ _ _ _]
      tunnel: [w404 w433 w499 w551 w558 w568 w580 w594 w620] -> w385
      tunnel: w384 -> [w414 w436 w502 w551 w558 w568 w580 w594 w620]
      tunnel: w383 -> [w408 w435 w500 w550 w557 w567 w579 w593 w619]
      tunnel: [w407 w432 w498 w550 w557 w567 w579 w593 w619] -> w382
      tunnel: "array size" -> [w406 w434 w501 _ _ _ _ _ _]
      frame "idle", Default {
        n218 = local read "threshold"() -> (w426:i32)
        n219 = call "tm_getnextframe_a.vi"("error in (no error)"=w424, "Buffer"=w421, "Handle in"=w425) -> ("error out"=w422:errorcluster, "Data"=w416:u16[][], "Handle out"=w423:u32)  [unwired: 6 in]
        n220 = local read "dark?"() -> (w427:bool)
        n221 = local read "count?"() -> (w417:bool)
        n222 = case shown="True" w427 {
          tunnel: [w428 w431] -> w418
          tunnel: w416 -> [w428 w430]
          tunnel: w420 -> [_ w429]
          frame False {
          }
          frame True {
            n223 = Subtract(x=w430, y=w429) -> (x-y=w431:dbl[][])
          }
        }
        n224 = call "filtr_b.vi"("count?"=w417, "threshold"=w426, "input array"=w418) -> ("output array"=w415:dbl[][])  [unwired: 8 in]
        n225 = Add Array Elements(numeric array=w415) -> (sum=w413:dbl)
        n226 = call "ringbuffer.vi"("new val"=w413, "index in"=w408, "array size"=w406, "array in"=w414) -> ("index out"=w407:i32, "array out"=w404:dbl[])  [unwired: 6 in]
        n227 = local write "live"(w415) -> ()
        n228 = local write "Waveform Chart"(w413) -> ()
        n229 = call <vilib>:"Std Deviation and Variance.vi"("X"=w404) -> ("mean"=w409:dbl, "standard deviation"=w412:dbl)  [unwired: 1 in, 1 out]
        n230 = Divide(x=w412, y=w409) -> (x/y=w411:dbl)
        n231 = Multiply(x=w411, y=100.0) -> (x*y=w405:dbl)
        n232 = local write "signal noise-o-meter"(w405) -> ()
      }
      frame "snap" {
        n233 = Dequeue Element(queue=w442) -> ()  [unwired: 2 in, 4 out]
        n234 = local read "avg[t] acc[f]"() -> (w441:bool)
        n235 = local read "threshold"() -> (w449:i32)
        n236 = local read "frames"() -> (w448:i32)
        n237 = local read "count?"() -> (w440:bool)
        n238 = local read "dark?"() -> (w450:bool)
        n239 = for {
          N: w448 -> [w469]
          tunnel: w450 -> [w483]
          tunnel: w446 -> [w481]
          tunnel: w445 -> [w482]
          tunnel: w449 -> [w475]
          tunnel: [w479] -> w439
          shift-right: [w478] -> w444
          shift-left: w447 -> [w480]
          tunnel: w443 -> [w474]
          shift-right: [w468] -> w437
          shift-left: w446 -> [w472]
          tunnel: w441 -> [w473]
          tunnel: w440 -> [w471]
          shift-right: [w460] -> w433
          shift-left: w436 -> [w461]
          tunnel: w434 -> [w458]
          shift-right: [w457] -> w432
          shift-left: w435 -> [w459]
          shift-right: [w452] -> _
          shift-left: _ -> [w453]
          i -> [w470]
          stop <- "stop" stop-if-true
          n240 = call "tm_getnextframe_a.vi"("error in (no error)"=w480, "Buffer"=w481, "Handle in"=w482) -> ("error out"=w478:errorcluster, "Data"=w477:u16[][], "Handle out"=w479:u32)  [unwired: 6 in]
          n241 = Divide(x=w470, y=w469) -> (x/y=w466:dbl)
          n242 = case shown="True" w483 {
            tunnel: [w494 w497] -> w476
            tunnel: w477 -> [w494 w496]
            tunnel: w474 -> [_ w495]
            frame False {
            }
            frame True {
              n243 = Subtract(x=w496, y=w495) -> (x-y=w497:dbl[][])
            }
          }
          n244 = local write "Slide"(w466) -> ()
          n245 = Tick Count (ms)() -> (millisecond timer value=w452:u32)
          n246 = call "filtr_b.vi"("count?"=w471, "threshold"=w475, "input array"=w476) -> ("output array"=w467:dbl[][])  [unwired: 8 in]
          n247 = Subtract(x=w452, y=w453) -> (x-y=w451:u32)
          n248 = Add Array Elements(numeric array=w467) -> (sum=w456:dbl)
          n249 = call "ringbuffer.vi"("new val"=w456, "index in"=w459, "array size"=w458, "array in"=w461) -> ("index out"=w457:i32, "array out"=w460:dbl[])  [unwired: 6 in]
          n250 = call <vilib>:"Std Deviation and Variance.vi"("X"=w460) -> ("mean"=w462:dbl, "standard deviation"=w464:dbl)  [unwired: 1 in, 1 out]
          n251 = local write "live"(w467) -> ()
          n252 = local write "Waveform Chart"(w456) -> ()
          n253 = Divide(x=w464, y=w462) -> (x/y=w455:dbl)
          n254 = case shown="True" w473 {
            tunnel: w472 -> [w486 w493]
            tunnel: w467 -> [w485 w491]
            tunnel: [w484 w487] -> w468
            tunnel: w470 -> [_ w488]
            frame False {
              n255 = Add(x=w486, y=w485) -> (x+y=w484:dbl[][])
            }
            frame True {
              n256 = Multiply(x=w493, y=w488) -> (x*y=w492:dbl[][])
              n257 = Increment(x=w488) -> (x+1=w489:i32)
              n258 = Add(x=w492, y=w491) -> (x+y=w490:dbl[][])
              n259 = Divide(x=w490, y=w489) -> (x/y=w487:dbl[][])
            }
          }
          n260 = local write "x-y"(w451) -> ()
          n261 = local write "captured"(w468) -> ()
          n262 = Multiply(x=w455, y=100.0) -> (x*y=w454:dbl)
          n263 = local write "signal noise-o-meter"(w454) -> ()
        }
        n264 = local write "captured"(w437) -> ()
        n265 = Enqueue Element(queue=w438, element=w437) -> ()  [unwired: 2 in, 3 out]
      }
      frame "snap_I" {
        n266 = Dequeue Element(queue=w507) -> ()  [unwired: 2 in, 4 out]
        n267 = local read "threshold"() -> (w518:i32)
        n268 = local read "frames"() -> (w517:i32)
        n269 = local read "count?"() -> (w516:bool)
        n270 = local read "dark?"() -> (w519:bool)
        n271 = for {
          N: w517 -> [w533]
          tunnel: w519 -> [w545]
          tunnel: w510 -> [w543]
          tunnel: w515 -> [w544]
          tunnel: w518 -> [w537]
          tunnel: [w541] -> w511
          shift-right: [w540] -> w512
          shift-left: w514 -> [w542]
          tunnel: w513 -> [w536]
          tunnel: w516 -> [w535]
          tunnel: [w531] -> w509 mode=indexing
          shift-right: [w523] -> w499
          shift-left: w502 -> [w524]
          tunnel: w501 -> [w522]
          shift-right: [w520] -> w498
          shift-left: w500 -> [w521]
          i -> [w534]
          n272 = call "tm_getnextframe_a.vi"("error in (no error)"=w542, "Buffer"=w543, "Handle in"=w544) -> ("error out"=w540:errorcluster, "Data"=w539:u16[][], "Handle out"=w541:u32)  [unwired: 6 in]
          n273 = call "ringbuffer.vi"("index in"=w521, "array size"=w522, "array in"=w524) -> ("index out"=w520:i32, "array out"=w523:dbl[])  [unwired: 7 in]
          n274 = Divide(x=w534, y=w533) -> (x/y=w532:dbl)
          n275 = case shown="True" w545 {
            tunnel: [w546 w549] -> w538
            tunnel: w539 -> [w546 w548]
            tunnel: w536 -> [_ w547]
            frame False {
            }
            frame True {
              n276 = Subtract(x=w548, y=w547) -> (x-y=w549:dbl[][])
            }
          }
          n277 = local write "Slide"(w532) -> ()
          n278 = call <vilib>:"Std Deviation and Variance.vi"("X"=w523) -> ("mean"=w525:dbl, "standard deviation"=w528:dbl)  [unwired: 1 in, 1 out]
          n279 = call "filtr_b.vi"("count?"=w535, "threshold"=w537, "input array"=w538) -> ("output array"=w530:dbl[][])  [unwired: 8 in]
          n280 = Divide(x=w528, y=w525) -> (x/y=w527:dbl)
          n281 = local write "live"(w530) -> ()
          n282 = Multiply(x=w527, y=100.0) -> (x*y=w529:dbl)
          n283 = local write "signal noise-o-meter"(w529) -> ()
          n284 = Add Array Elements(numeric array=w530) -> (sum=w531:dbl)
          n285 = local write "Waveform Chart"(w531) -> ()
        }
        n286 = call <vilib>:"Std Deviation and Variance.vi"("X"=w509) -> ("mean"=w506:dbl, "standard deviation"=w505:dbl)  [unwired: 1 in, 1 out]
        n287 = Format Into String(format string="%.6e;%.6e", w506, w505) -> (resulting string=w504:string)  [unwired: 2 in, 1 out]
        n288 = Enqueue Element(queue=w508, element=w504) -> ()  [unwired: 2 in, 3 out]
      }
      frame "dark" {
        n289 = Dequeue Element(queue=w556) -> ()  [unwired: 2 in, 4 out]
        n290 = local read "captured"() -> (w552:dbl[][])
      }
      frame "dark_load" {
        n291 = Dequeue Element(queue=w566) -> ()  [unwired: 2 in, 4 out]
        n292 = String To Path(string=w562) -> (path=w561:path)
        n293 = Read from Binary File(5:dbl[][] [] ("all rows"), 11:w561) -> (2:w559:dbl[][])  [unwired: 4 in, 3 out]
        n294 = call-poly <vilib>:"Read From Spreadsheet File.vi"("file path (dialog if empty)"=w561) -> ()  [unwired: 6 in, 5 out]
      }
      frame "release" {
        n295 = call "tm_stopcapture.vi"("error in (no error)"=w574, "Handle in"=w575) -> ("error out"=w572:errorcluster, "Handle out"=w573:u32)  [unwired: 8 in]
        n296 = Dequeue Element(queue=w578) -> ()  [unwired: 2 in, 4 out]
        n297 = call "tm_closecamera.vi"("error in (no error)"=w572, "Handle in"=w573) -> ("error out"=w571:errorcluster)  [unwired: 9 in]
        n298 = call "tm_deinitialize.vi"("error in (no error)"=w571) -> ("error out"=w570:errorcluster)  [unwired: 10 in]
      }
      frame "init" {
        n299 = Dequeue Element(queue=w581) -> ()  [unwired: 2 in, 4 out]
        n300 = call "tm_initialize.vi"() -> ("error out"=w587:errorcluster)  [unwired: 8 in, 3 out]
        n301 = call "tm_opencamera.vi"("error in (no error)"=w587, "Camera Index"=u32 0) -> ("error out"=w586:errorcluster, "Handle out"=w584:u32)  [unwired: 7 in, 1 out]
      }
      frame "set" {
        w606 = 1 items=["Snap", "Sequence"] ("Capture mode")
        w608 = u32 4215968 items=["BINNING"=4215968, "BITS PER CHANNEL"=2, "ACTIVE VIEW INDEX"=3, "CCD MODE"=4, "SENSOR MODE"=5, "READOUT MODE"=6, "EXPOSURE TIME"=7, "CONTRAST GAIN"=8, "CONTRAST OFFSET"=9, "LIGHT MODE"=10, "SENSITIVITY"=11, "WHITE BALANCE"=12, "PHOTON IMAGING MODE"=13, "HIGH DYNAMIC RANGE MODE"=14, "TRIGGER SOURCE"=15, "TRIGGER ACTIVE"=16, "TRIGGER MODE"=17, "TRIGGER POLARITY"=18, "TRIGGER GLOBAL EXPOSURE"=19, "FIRST TRIGGER BEHAVIOR"=20, "TRIGGER TIMES"=21, "OUTPUT TRIGGER POLARITY"=22, "OUTPUT TRIGGER DELAY"=23, "OUTPUT TRIGGER PERIOD"=24, "TEMPERATURE"=25, "TEMPERATURE TARGET"=26, "SENSOR COOLER FAN"=27, "MECHANICAL SHUTTER"=28, "BACK FOCUS POSITION"=29, "FRAMEBUNDLE MODE"=30, "FRAMEBUNDLE NUMBER"=31, "LINEBUNDLE HEIGHT"=32, "TRIGGER CONNECTOR"=33, "IMAGE PIXEL TYPE"=34, "OUTPUT TRIGGER KIND"=35, "READOUT DIRECTION"=36, "CHANNEL SYNC"=37] ("Parameter")
        w612 = u32 7 items=["BINNING"=4215968, "BITS PER CHANNEL"=2, "ACTIVE VIEW INDEX"=3, "CCD MODE"=4, "SENSOR MODE"=5, "READOUT MODE"=6, "EXPOSURE TIME"=7, "CONTRAST GAIN"=8, "CONTRAST OFFSET"=9, "LIGHT MODE"=10, "SENSITIVITY"=11, "WHITE BALANCE"=12, "PHOTON IMAGING MODE"=13, "HIGH DYNAMIC RANGE MODE"=14, "TRIGGER SOURCE"=15, "TRIGGER ACTIVE"=16, "TRIGGER MODE"=17, "TRIGGER POLARITY"=18, "TRIGGER GLOBAL EXPOSURE"=19, "FIRST TRIGGER BEHAVIOR"=20, "TRIGGER TIMES"=21, "OUTPUT TRIGGER POLARITY"=22, "OUTPUT TRIGGER DELAY"=23, "OUTPUT TRIGGER PERIOD"=24, "TEMPERATURE"=25, "TEMPERATURE TARGET"=26, "SENSOR COOLER FAN"=27, "MECHANICAL SHUTTER"=28, "BACK FOCUS POSITION"=29, "FRAMEBUNDLE MODE"=30, "FRAMEBUNDLE NUMBER"=31, "LINEBUNDLE HEIGHT"=32, "TRIGGER CONNECTOR"=33, "IMAGE PIXEL TYPE"=34, "OUTPUT TRIGGER KIND"=35, "READOUT DIRECTION"=36, "CHANNEL SYNC"=37] ("Parameter")
        n302 = Dequeue Element(queue=w600) -> ()  [unwired: 2 in, 4 out]
        n303 = call "tm_stopcapture.vi"("error in (no error)"=w618, "Handle in"=w616) -> ("error out"=w617:errorcluster, "Handle out"=w615:u32)  [unwired: 8 in]
        n304 = call "tm_unpreparecapture.vi"("error in (no error)"=w617, "Handle in"=w615) -> ("error out"=w614:errorcluster, "Handle out"=w613:u32)  [unwired: 8 in]
        n305 = call "tm_setparameter.vi"("error in (no error)"=w614, "Value in"="exp time [s]", "Parameter"=w612, "Handle in"=w613) -> ("error out"=w609:errorcluster, "Handle out"=w610:u32)  [unwired: 6 in]
        n306 = call "tm_setparameter.vi"("error in (no error)"=w609, "Value in"="binning", "Parameter"=w608, "Handle in"=w610) -> ("error out"=w590:errorcluster, "Handle out"=w591:u32)  [unwired: 6 in]
        n307 = call "tm_preparecapture.vi"("error in (no error)"=w590, "Frames"=1, "Capture mode"=w606, "Handle in"=w591) -> ("error out"=w603:errorcluster, "Buffer Info"=w602:T5, "Handle out"=w604:u32)  [unwired: 4 in, 1 out]
        n308 = call "tm_startcapture_b.vi"("error in (no error)"=w603, "Handle in"=w604) -> ("error out"=w588:errorcluster, "Handle out"=w589:u32)  [unwired: 8 in]
        n309 = Unbundle(w602) -> ("height"=w598:u32, "width"=w599:u32)  [unwired: 1 out]
        n310 = property on="live" class="IntGraph (strict)"("XScale.Minimum"=0.0 ("X Scale.Range:Minimum"), "XScale.Maximum"=w598, "YScale.Minimum"=0.0 ("Y Scale.Range:Minimum"), "YScale.Maximum"=w599) -> ()  [unwired: 2 in, 2 out]
        n311 = Initialize Array(u16 0 ("element"), w598, w599) -> (w601:u16[][])
      }
      frame "close" {
        n312 = Release Queue(queue=w626) -> ()  [unwired: 2 in, 3 out]
      }
    }
  }
  n313 = while {
    tunnel: w10 -> [w635]
    shift-right: [w633] -> _
    shift-left: _ -> [w632]
    shift-right: [w630] -> _
    shift-left: 0 -> [w631]
    shift-right: [w629] -> _
    shift-left: _ -> [w628]
    tunnel: w1 -> [w627]
    stop <- w634 stop-if-true
    # "ISEG"
    n314 = Preview Queue Element(queue=w635, timeout in ms (-1)=w631) -> (element=w639:string)  [unwired: 1 in, 3 out]
    n315 = Match Pattern(string=w639, regular expression=":") -> (before substring=w637:string, after substring=w636:string)  [unwired: 1 in, 2 out]
    n316 = case shown="\"idle\", Default" w637 {
      tunnel: w636 -> [_ w655 _ _ _]
      tunnel: w635 -> [_ w667 w709 w713 w717]
      tunnel: [_ _ _ _ TRUE] -> w634
      tunnel: [w644 w661 w707 w712 w714] -> w633
      tunnel: w632 -> [w646 w665 _ _ w714]
      tunnel: [0 _ _ _ _] -> w630
      tunnel: [w645 w662 T6 {"VISA Resource Name"="", "FP Notation"=FALSE, "Maximum Voltage"=0, "Maximum Current"=0} ("VISA Session Out") w710 w715] -> w629
      tunnel: w628 -> [w647 w666 w708 _ w715]
      tunnel: w627 -> [_ w650 _ _ _]
      frame "idle", Default {
        n317 = local read "Channel (A)"() -> (w648:enum16{"A", "B"})
        n318 = call "iseg NHQ xxx GetActualVoltage.vi"("error in (no error)"=w646, "Channel (A)"=w648, "VISA Session"=w647) -> ("error out"=w644:errorcluster, "Voltage"=w642:dbl, "VISA Session Out"=w645:T6)  [unwired: 5 in, 1 out]
        n319 = Round To Nearest(number=w642) -> (nearest integer value=w641:dbl)
        n320 = node(w642) -> (→"Actual Voltage":dbl[unit])
        n321 = Absolute Value(x=w641) -> (abs(x)=w640:dbl)
        n322 = local write "meas_voltage"(w640) -> ()
      }
      frame "set" {
        n323 = local read "Channel (A)"() -> (w658:enum16{"A", "B"})
        n324 = Dequeue Element(queue=w667) -> ()  [unwired: 2 in, 4 out]
        n325 = Match Pattern(string=w655, regular expression=":") -> (before substring=w654:string, after substring=w653:string)  [unwired: 1 in, 2 out]
        n326 = Fract/Exp String To Number(string=w654) -> (number=w657:dbl)  [unwired: 3 in, 1 out]
        n327 = call "iseg NHQ xxx SetNominalVoltage.vi"("error in (no error)"=w665, "Voltage (0 V)"=w657, "Channel (A)"=w658, "VISA Session"=w666) -> ("error out"=w668:errorcluster, "VISA Session Out"=w669:T6)  [unwired: 6 in]
        n328 = Equal?(x=w653, y="wait") -> (x = y?=w651:bool)
        n329 = call "iseg NHQ xxx StartVoltageChange.vi"("error in (no error)"=w668, "Channel (A)"=w658, "VISA Session"=w669) -> ("error out"=w663:errorcluster, "VISA Session Out"=w664:T6)  [unwired: 6 in, 1 out]
        n330 = case shown="True" w651 {
          tunnel: [w671 w681] -> w662
          tunnel: [w670 w673] -> w661
          tunnel: w664 -> [w671 w680]
          tunnel: w663 -> [w670 w679]
          tunnel: w657 -> [_ w678]
          tunnel: "volt_threshold" -> [_ w677]
          tunnel: "volt_timeout" -> [_ w676]
          tunnel: w658 -> [_ w675]
          tunnel: w650 -> [_ w674]
          frame False {
          }
          frame True {
            n331 = Tick Count (ms)() -> (millisecond timer value=w682:u32)
            n332 = while {
              shift-right: [w703] -> w681
              shift-left: w680 -> [w705]
              shift-right: [w690] -> w673
              shift-left: w679 -> [w704]
              tunnel: w675 -> [w702]
              tunnel: w677 -> [w699]
              tunnel: w682 -> [w697]
              tunnel: w676 -> [w695]
              tunnel: w678 -> [w694]
              tunnel: [w685] -> w672
              stop <- w691 stop-if-true
              n333 = Tick Count (ms)() -> (millisecond timer value=w698:u32)
              n334 = call "iseg NHQ xxx GetActualVoltage.vi"("error in (no error)"=w704, "Channel (A)"=w702, "VISA Session"=w705) -> ("error out"=w690:errorcluster, "Voltage"=w683:dbl, "VISA Session Out"=w703:T6)  [unwired: 5 in, 1 out]
              n335 = Absolute Value(x=w683) -> (abs(x)=w693:dbl)
              n336 = node(w683) -> (w684:dbl[unit])
              n337 = Subtract(x=w698, y=w697) -> (x-y=w696:u32)
              n338 = Subtract(x=w693, y=w694) -> (x-y=w701:dbl)
              n339 = local write "Actual Voltage"(w684) -> ()
              n340 = Absolute Value(x=w701) -> (abs(x)=w700:dbl)
              n341 = Greater?(x=w696, y=w695) -> (0:w689:bool)
              n342 = Less?(x=w700, y=w699) -> (x < y?=w692:bool)
              n343 = Or(x=w690, y=w689) -> (x .or. y?=w688:bool)
              n344 = Compound Arithmetic op=OR(w690, w692, w689) -> (w691:bool)
              n345 = Select(t="fail" ("element"), s=w688, f="done" ("element")) -> (s? t:f=w685:string)
            }
            n346 = Enqueue Element(queue=w674, element=w672) -> ()  [unwired: 2 in, 3 out]
          }
        }
      }
      frame "release" {
        n347 = Dequeue Element(queue=w709) -> ()  [unwired: 2 in, 4 out]
        n348 = call "iseg NHQ xxx Close.vi"("VISA session"=w708) -> ("error out"=w707:errorcluster)  [unwired: 14 in]
      }
      frame "init" {
        n349 = Dequeue Element(queue=w713) -> ()  [unwired: 2 in, 4 out]
        n350 = call "iseg NHQ xxx Initialize.vi"("VISA resource name"="VISA ISEG") -> ("VISA Session Out"=w710:T6, "error out"=w712:errorcluster)  [unwired: 13 in]
      }
      frame "close" {
        n351 = Release Queue(queue=w717) -> ()  [unwired: 2 in, 3 out]
      }
    }
    "error out" <- w633
  }
  n352 = while {
    tunnel: w3 -> [w732]
    shift-right: [w722] -> _
    shift-left: errorcluster {"status"=FALSE, "code"=0, "source"=""} ("error constant") -> [w730]
    shift-right: [w724] -> _
    shift-left: _ -> [w729]
    shift-right: [w728] -> _
    shift-left: _ -> [w727]
    tunnel: w1 -> [w726]
    tunnel: w5 -> [w725]
    tunnel: [w725] -> w4
    shift-right: [w721] -> _
    shift-left: _ -> [w720]
    shift-right: [w719] -> _
    shift-left: _ -> [w718]
    stop <- w731 stop-if-true
    # "COHERENT"
    n353 = Preview Queue Element(queue=w732, timeout in ms (-1)=w729) -> (element=w736:string)  [unwired: 1 in, 3 out]
    n354 = Match Pattern(string=w736, regular expression=":") -> (before substring=w734:string, after substring=w733:string)  [unwired: 1 in, 2 out]
    n355 = case shown="\"start\"" w734 {
      tunnel: w733 -> [_ _ _ _ _ _]
      tunnel: w732 -> [_ w774 w820 w830 w838 w846]
      tunnel: [_ _ _ _ _ TRUE] -> w731
      tunnel: [w753 w768 w814 w828 w835 w843] -> w722
      tunnel: w730 -> [w755 w771 w816 _ w834 w843]
      tunnel: [0 _ _ _ _ _] -> w723
      tunnel: [w754 w769 w815 0 ("Meter Index") w836 w844] -> w728
      tunnel: w727 -> [w756 w772 w817 w826 _ w844]
      tunnel: w726 -> [_ w770 w819 _ _ _]
      tunnel: [w741 w762 w803 w825 w832 w842] -> w721
      tunnel: w720 -> [w745 w764 w808 w825 w832 w842]
      tunnel: [w743 w761 w806 w824 w831 w841] -> w719
      tunnel: w718 -> [w742 w763 w807 w824 w831 w841]
      frame "idle", Default {
        n356 = call "CH_LM Measurement Fetch Data.vi"("Meter Index"=w756, "error in (no error)"=w755) -> ("Meter Index"=w754:i32, "Data Array"=w752:T7[], "error out"=w753:errorcluster)  [unwired: 13 in, 2 out]
        n357 = Index Array(array=w752) -> (element=w751:T7)  [unwired: 1 in]
        n358 = Unbundle By Name(w751) -> ("Value"=w740:sgl)
        n359 = call "ringbuffer.vi"("new val"=w740, "index in"=w742, "array size"="array size 2", "array in"=w745) -> ("index out"=w743:i32, "array out"=w741:dbl[])  [unwired: 6 in]
        n360 = node(w740) -> (→"laser power" →"meas_power":sgl[unit])
        n361 = call <vilib>:"Std Deviation and Variance.vi"("X"=w741) -> ("mean"=w746:dbl, "standard deviation"=w749:dbl)  [unwired: 1 in, 1 out]
        n362 = Divide(x=w749, y=w746) -> (x/y=w748:dbl)
        n363 = Multiply(x=w748, y=100.0) -> (x*y=→"power noise-o-meter":dbl)
      }
      frame "start" {
        n364 = Dequeue Element(queue=w774) -> (queue out=w773:refnum<queue>)  [unwired: 2 in, 3 out]
        n365 = while {
          tunnel: w773 -> [w798]
          tunnel: w772 -> [w795]
          tunnel: w771 -> [w794]
          tunnel: [w793] -> w769
          tunnel: [w792] -> w768
          tunnel: w764 -> [w790]
          tunnel: w763 -> [w789]
          tunnel: [w782] -> w762
          tunnel: [w788] -> w761
          shift-right: [w777] -> w758
          shift-left: dbl[] [] -> [w780]
          stop <- w799 continue-if-true
          n366 = call "CH_LM Measurement Fetch Data.vi"("Meter Index"=w795, "error in (no error)"=w794) -> ("Meter Index"=w793:i32, "Data Array"=w797:T7[], "error out"=w792:errorcluster)  [unwired: 13 in, 2 out]
          n367 = local read "array size 2"() -> (w781:i32)
          n368 = Index Array(array=w797) -> (element=w796:T7)  [unwired: 1 in]
          n369 = Dequeue Element(queue=w798, timeout in ms (-1)=0) -> (element=w801:string)  [unwired: 1 in, 3 out]
          n370 = Equal?(x=w801, y="") -> (x = y?=w799:bool)
          n371 = Unbundle By Name(w796) -> ("Value"=w778:sgl)
          n372 = call "ringbuffer.vi"("new val"=w778, "index in"=w789, "array size"=w781, "array in"=w790) -> ("index out"=w788:i32, "array out"=w782:dbl[])  [unwired: 6 in]
          n373 = call <vilib>:"Std Deviation and Variance.vi"("X"=w782) -> ("mean"=w783:dbl, "standard deviation"=w786:dbl)  [unwired: 1 in, 1 out]
          n374 = Build Array (concatenate)(w780, w778) -> (w777:dbl[])
          n375 = Divide(x=w786, y=w783) -> (x/y=w785:dbl)
          n376 = call <vilib>:"Std Deviation and Variance.vi"("X"=w777) -> ("mean"=w776:dbl)  [unwired: 1 in, 2 out]
          n377 = node(w778) -> (w779:sgl[unit])
          n378 = local write "laser power"(w779) -> ()
          n379 = Multiply(x=w785, y=100.0) -> (x*y=w787:dbl)
          n380 = local write "power noise-o-meter"(w787) -> ()
          n381 = node(w776) -> (w775:dbl[unit])
          n382 = local write "meas_power"(w775) -> ()
        }
        n383 = call <vilib>:"Std Deviation and Variance.vi"("X"=w758) -> ("mean"=w760:dbl, "standard deviation"=w766:dbl)  [unwired: 1 in, 1 out]
        n384 = Format Into String(format string="%.6e;%.6e", w760, w766) -> (resulting string=w765:string)  [unwired: 2 in, 1 out]
        n385 = Enqueue Element(queue=w770, element=w765) -> ()  [unwired: 2 in, 3 out]
      }
      frame "snap" {
        n386 = Dequeue Element(queue=w820) -> ()  [unwired: 2 in, 4 out]
        n387 = call "CH_LM Measurement Fetch Data.vi"("Meter Index"=w817, "error in (no error)"=w816) -> ("Meter Index"=w815:i32, "Data Array"=w822:T7[], "error out"=w814:errorcluster)  [unwired: 13 in, 2 out]
        n388 = local read "array size 2"() -> (w805:i32)
        n389 = Index Array(array=w822) -> (element=w821:T7)  [unwired: 1 in]
        n390 = Unbundle By Name(w821) -> ("Value"=w804:sgl)
        n391 = call "ringbuffer.vi"("new val"=w804, "index in"=w807, "array size"=w805, "array in"=w808) -> ("index out"=w806:i32, "array out"=w803:dbl[])  [unwired: 6 in]
        n392 = call <vilib>:"Std Deviation and Variance.vi"("X"=w803) -> ("mean"=w802:dbl, "standard deviation"=w811:dbl)  [unwired: 1 in, 1 out]
        n393 = node(w804) -> (w813:sgl[unit])
        n394 = local write "laser power"(w813) -> ()
        n395 = Divide(x=w811, y=w802) -> (x/y=w810:dbl)
        n396 = Multiply(x=w810, y=100.0) -> (x*y=w812:dbl)
        n397 = local write "power noise-o-meter"(w812) -> ()
        n398 = Format Into String(format string="%.6e", w813) -> (resulting string=w818:string)  [unwired: 2 in, 1 out]
        n399 = Enqueue Element(queue=w819, element=w818) -> ()  [unwired: 2 in, 3 out]
      }
      frame "release" {
        n400 = Dequeue Element(queue=w830) -> ()  [unwired: 2 in, 4 out]
        n401 = call "CH_LM Measurement Abort.vi"("Meter Index"=w826) -> ("Meter Index"=w827:i32)  [unwired: 16 in, 2 out]
        n402 = call "CH_LM Close.vi"("Meter Index"=w827) -> ("error out"=w828:errorcluster)  [unwired: 16 in, 2 out]
      }
      frame "init" {
        n403 = Dequeue Element(queue=w838) -> ()  [unwired: 2 in, 4 out]
        n404 = flat-sequence {
          tunnel: w834 -> [w840]
          tunnel: [w840] -> w833
          frame #0 {
            n405 = Wait (ms)(milliseconds to wait=u32 1000) -> ()  [unwired: 1 out]
          }
        }
        n406 = call "CH_LM Measurement Initiate.vi"("Meter Index"=0, "error in (no error)"=w833) -> ("Meter Index"=w836:i32, "error out"=w835:errorcluster)  [unwired: 15 in, 1 out]
      }
      frame "close" {
        n407 = Release Queue(queue=w846) -> ()  [unwired: 2 in, 3 out]
      }
    }
    "coherent" <- w722
    n408 = case shown="No Error" w722 {
      tunnel: [w737 -1] -> w724
      tunnel: w723 -> [w737 _]
      frame No Error {
      }
      frame Error {
      }
    }
  }
  n409 = Set Occurrence(w4) -> ()
